vi "op_Pedestal.vi"(0 "EQ folder path Refnum":refnum<vi>, 1 "HV enable button":bool caption="High Voltage enable", 2 "HV parameters Refnum":refnum<vi>, 3 "HV level Refnum":refnum<vi>, 4 "HV string Refnum":refnum<vi>, 5 "Stop ACQ button Refnum":refnum<vi>, 6 "ACQ Parameters (cluster)":T2={"Acquisition Mode"=0, "Pulse width"=0, "DTP period"=1, "Number of events"=4000} caption="Acquisition Parameters" {"Number of events" min=1; "DTP period" min=1; "Pulse width" items=["25 ns", "50 ns", "75 ns", "100 ns"]; "Acquisition Mode" items=["Normal", "Pedestal", "Test Pulse", "Test Pulse trigger & synchronous"]}, 7 "Events to acquire Refnum":refnum<vi>, 8 "error tick Refnum":refnum<vi>, 9 "ACQ events fets Refnum":refnum<vi>, 10 "Operation text Refnum":refnum<vi>, 11 "ACQ events fets A Refnum":refnum<vi>, 12 "Busy Refnum":refnum<vi>, 13 "ACQ events fets B Refnum":refnum<vi>, 14 "Addresses Cluster":T1={"ENA1"=FALSE, "IP address 1"="172.16.14.22", "ENA2"=FALSE, "IP address 2"="172.16.14.23"}, 15 "etapa# terminals refnums":T3, 17 "GbReg params":u8[](array[numeric])=[32, 32]) -> (23 "Folder path: acquisition reports":path=path "C:/VIPauto/Files/LayerID/Acquisition/yyyymmdd_hh-mm-ss_Leak#_HV#")   [LabVIEW 2015, in "VIPM2.lvlib"]
uses:
  VIPM2.lvlib
panel:
  out "Chip ID list 2":u32[](array[numeric]) format="%.0x"
  out "Layer ID list 2 (ordered)":u32[](array[numeric]) format="%.0x"
  out "All ID list 2":u32[](array[numeric]) format="%.0x"
  out "All ID list 1":u32[](array[numeric]) format="%.0x"
  out "Layer ID list 1 (ordered)":u32[](array[numeric]) format="%.0x"
  out "Chip ID list 1":u32[](array[numeric]) format="%.0x"
  # "Operation: ACQuisition Pedestal with HV (refnums)"
  # "Analog Vref low"
  # "Gb THLD"
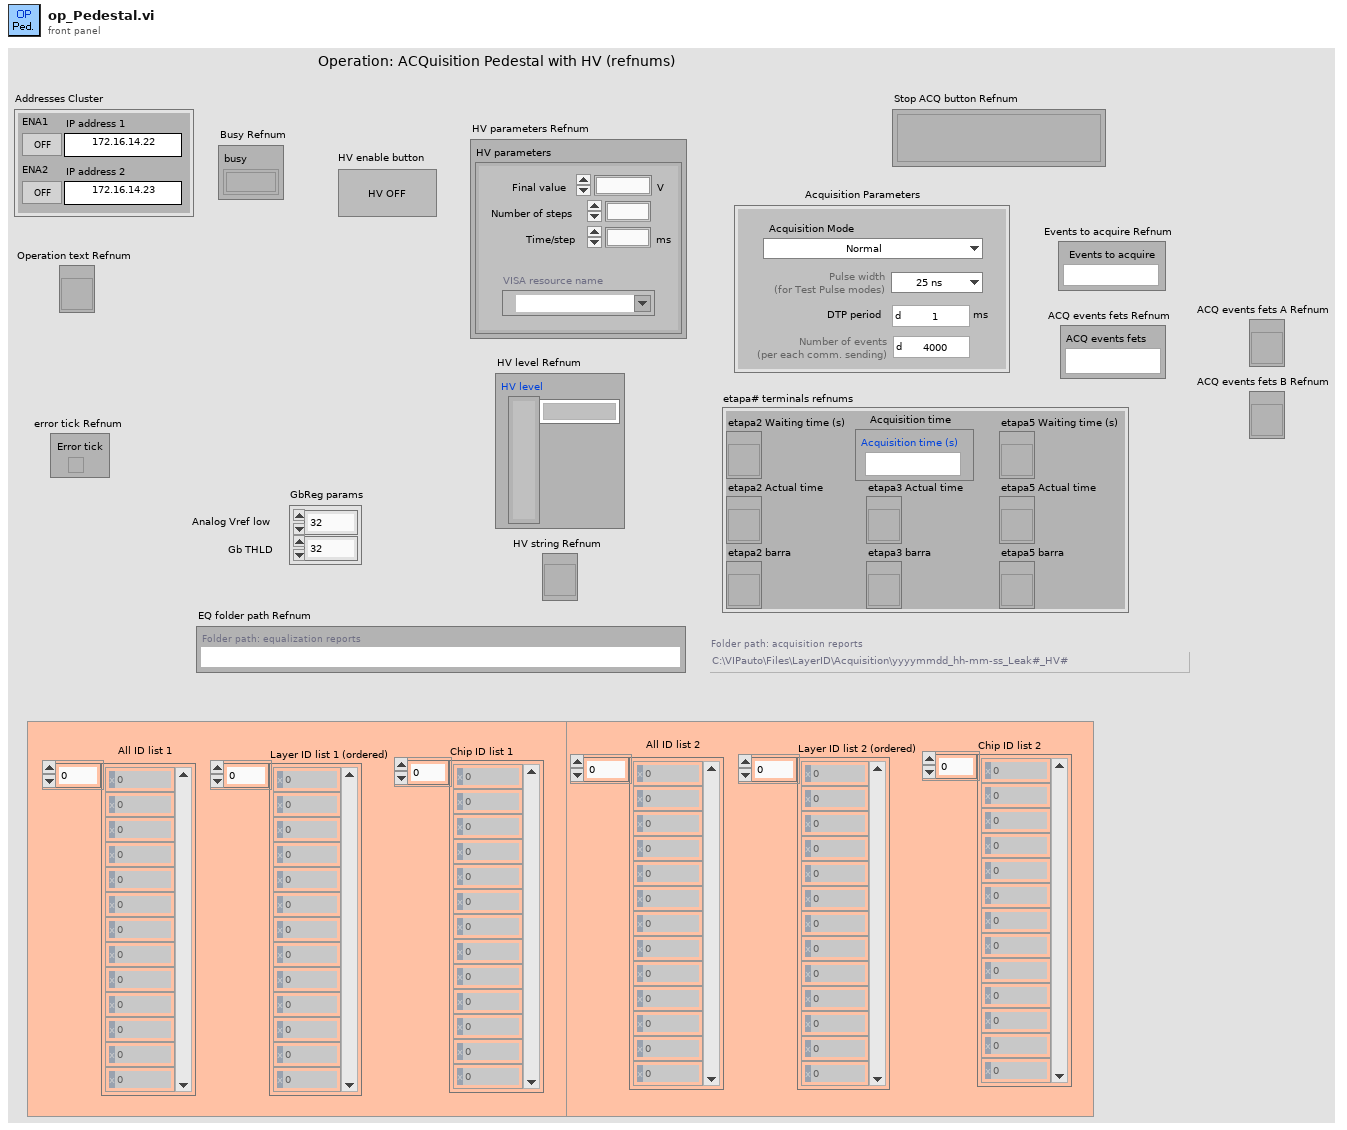
[diagram p1: front panel]
types:
  T1 = cluster{"ENA1":bool, "IP address 1":string, "ENA2":bool, "IP address 2":string}
  T2 = cluster{"Acquisition Mode":u32, "Pulse width":u32, "DTP period":u32, "Number of events":u32}
  T3 = cluster{"etapa2 Waiting time (s)":refnum<vi>, "etapa2 Actual time":refnum<vi>, "etapa2 barra":refnum<vi>, "etapa3 Actual time":refnum<vi>, "etapa3 barra":refnum<vi>, "etapa5 Waiting time (s)":refnum<vi>, "etapa5 Actual time":refnum<vi>, "etapa5 barra":refnum<vi>, "Acquisition time":refnum<vi>}
  T4 = enum8{"Enabled", "Disabled", "Disabled and Grayed Out"}
  T5 = cluster{"Final value":i16, "Number of steps":u8, "Time/step":u16, "Output Off Behavior":u16, "VISA resource name":refnum<visa-resource-name>}
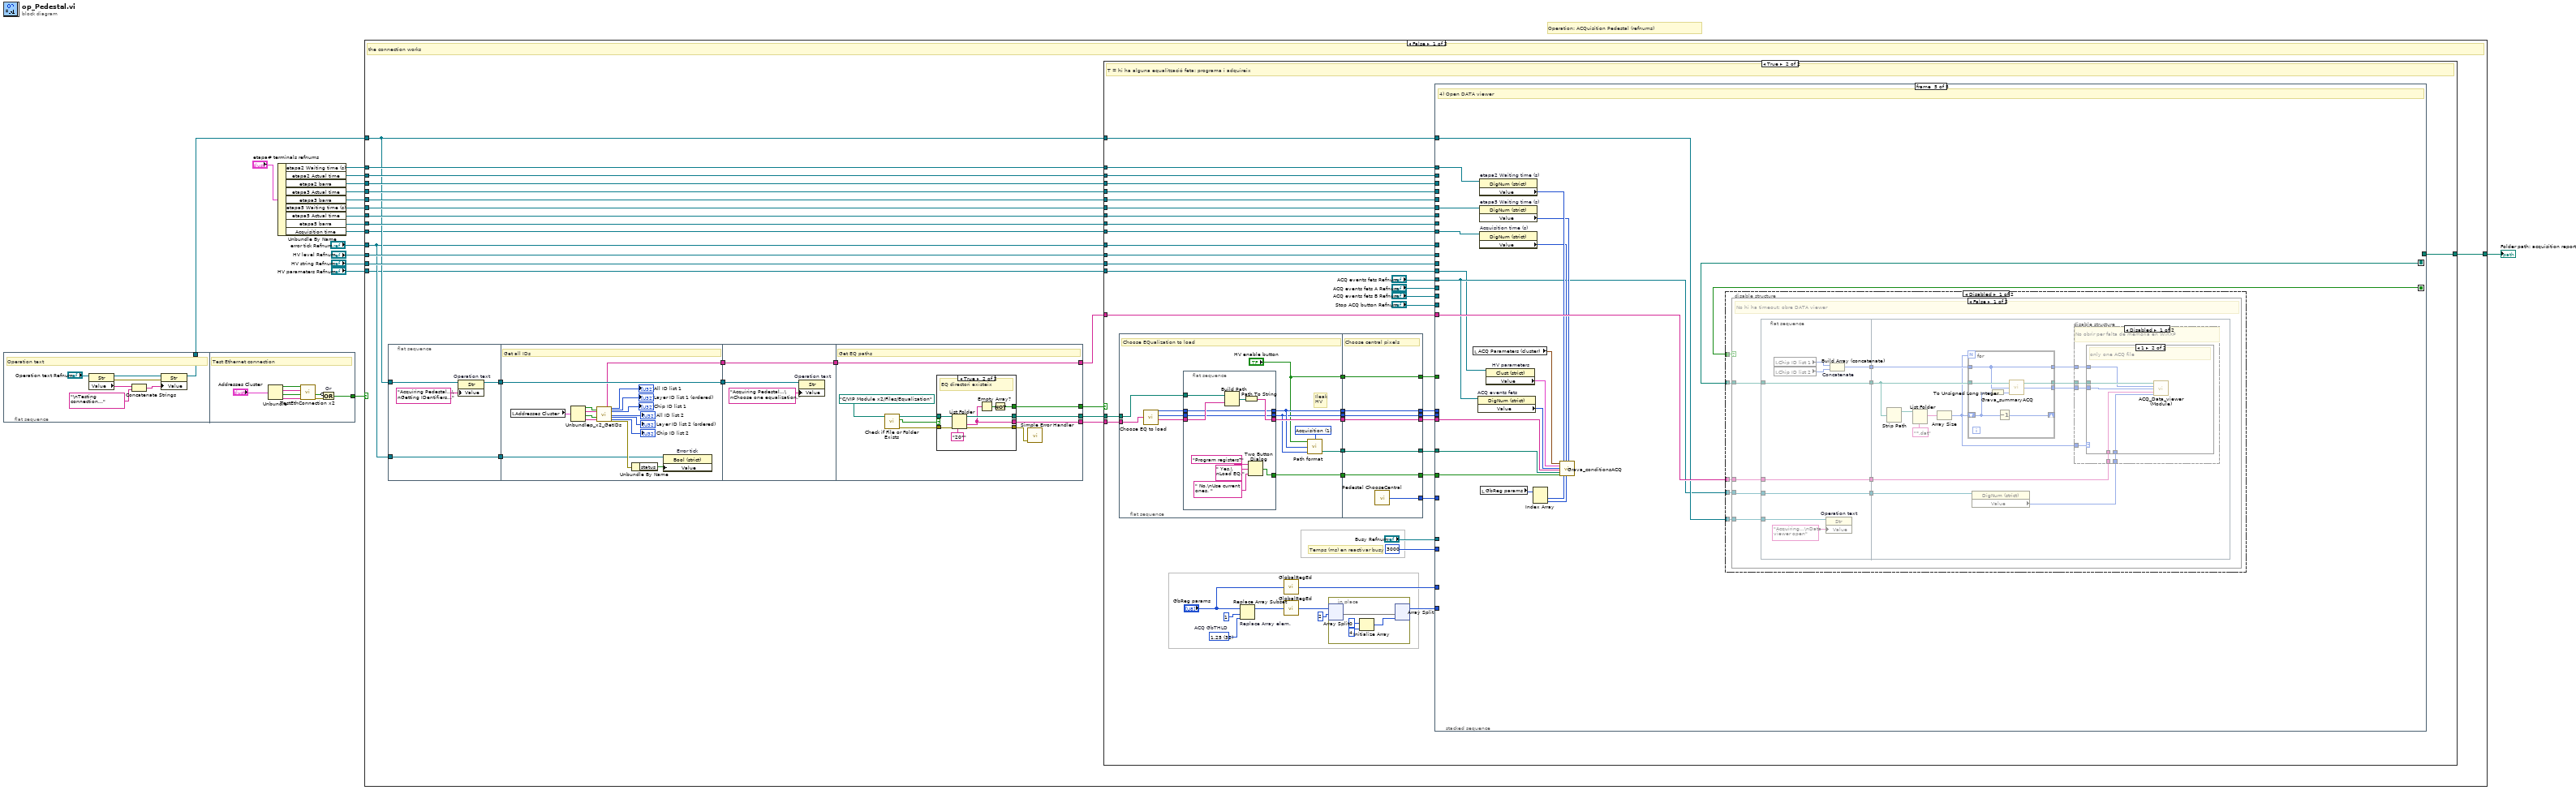
[diagram p0: block diagram]
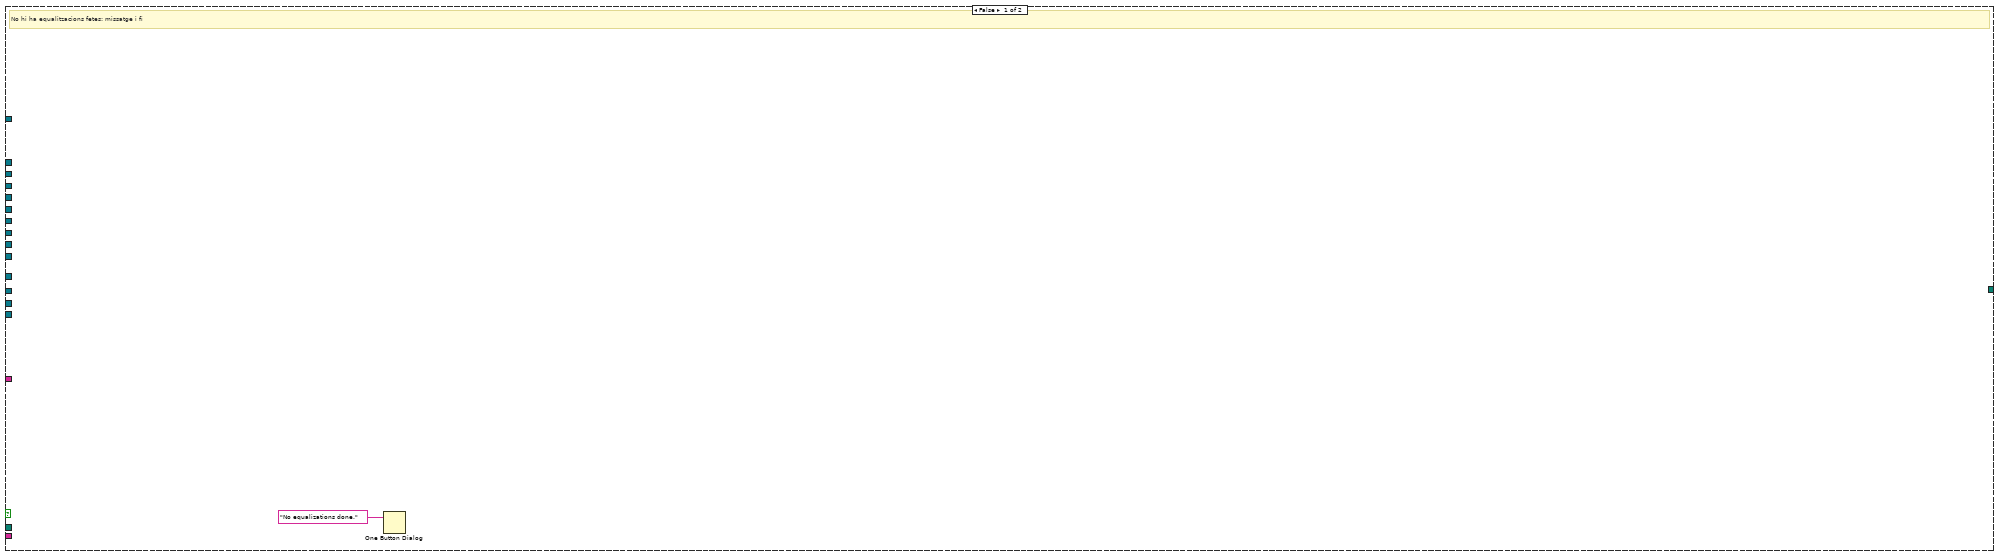
[diagram p3: hidden frame]
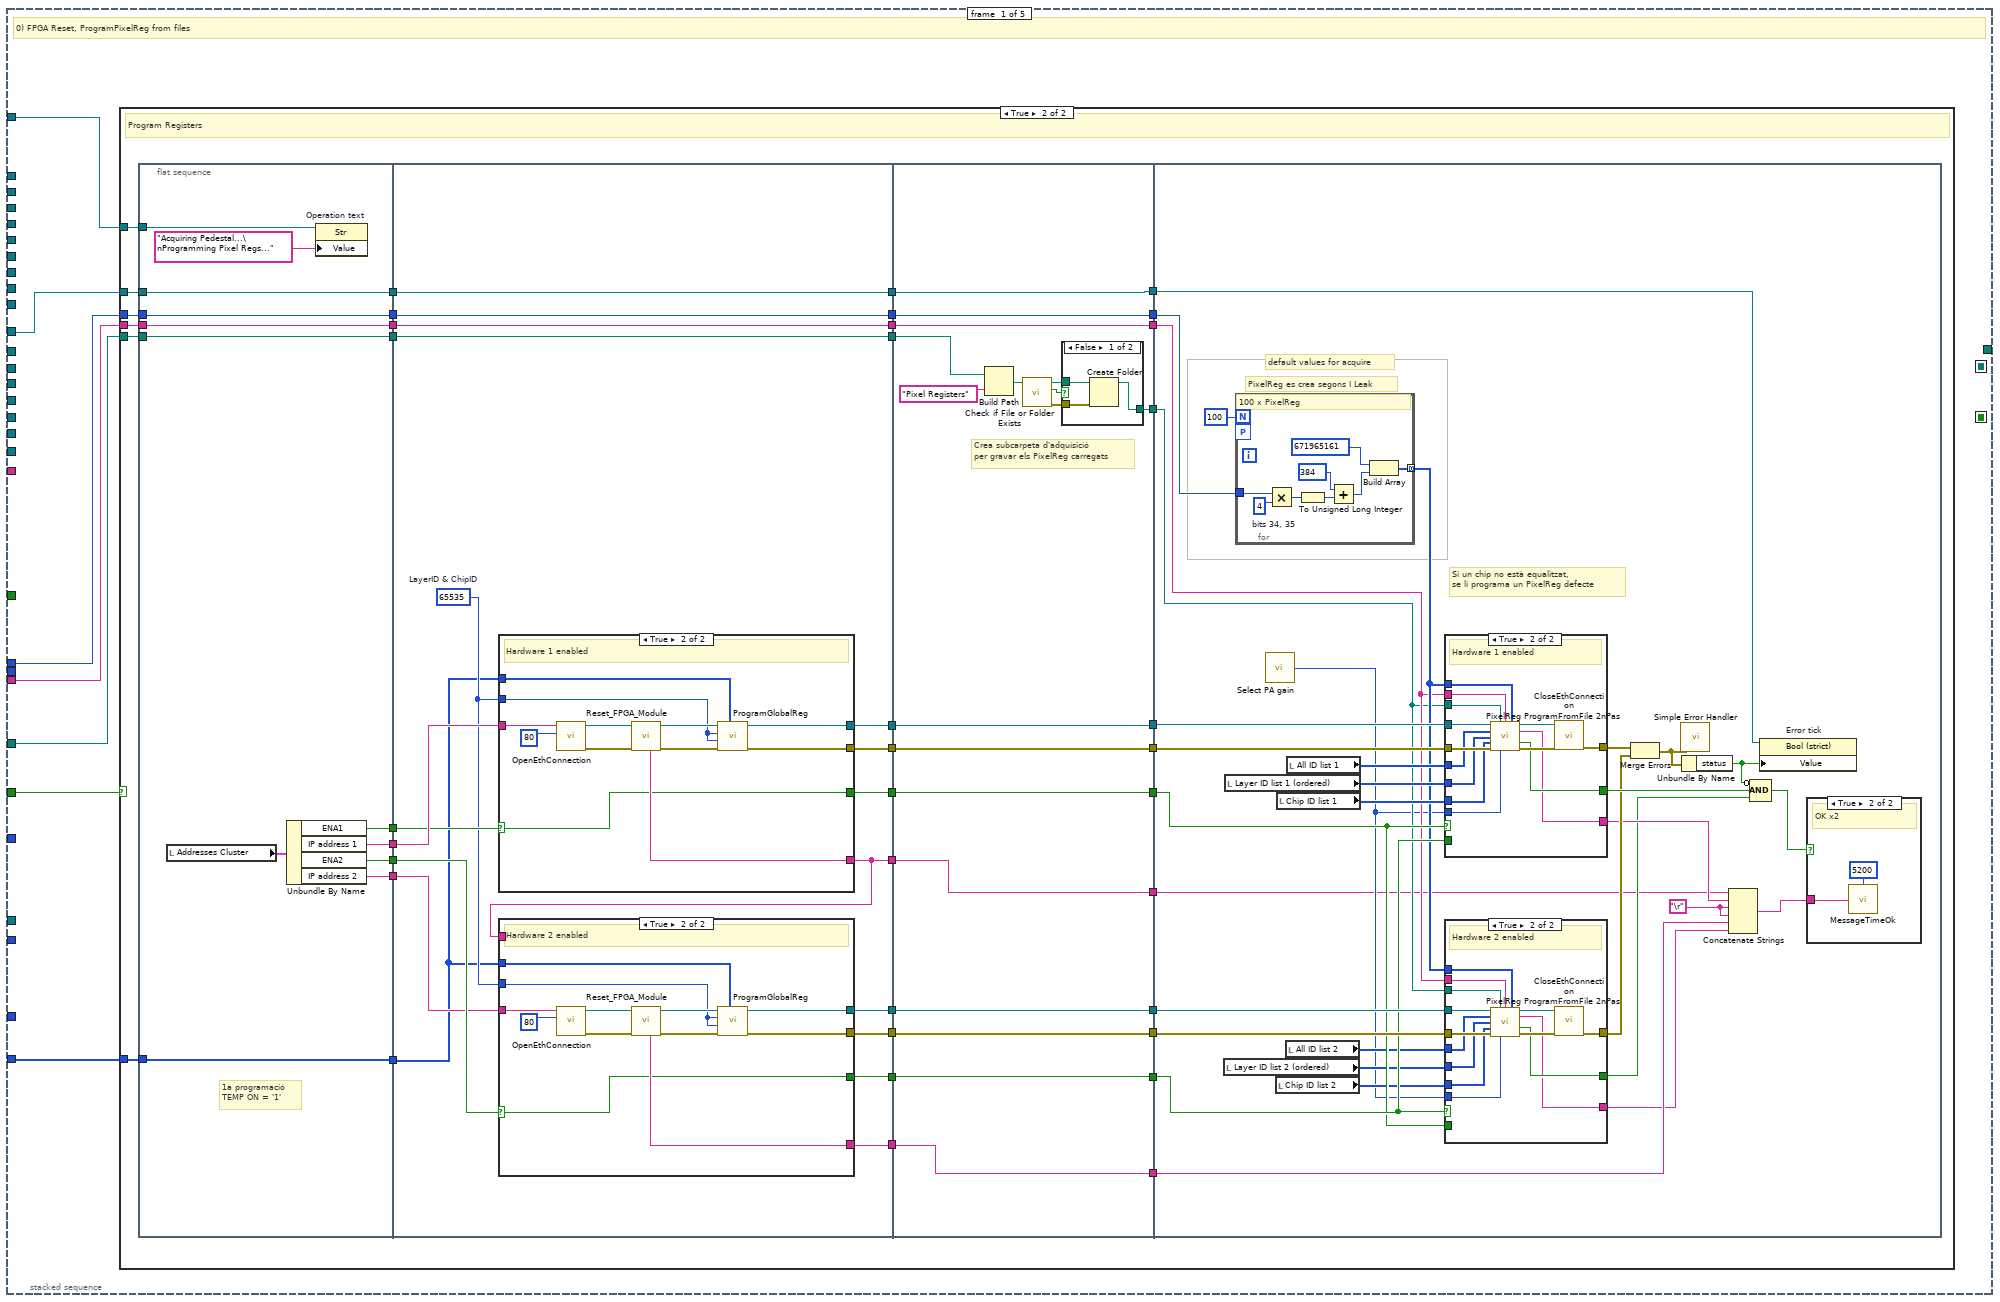
[diagram p4: hidden frame]
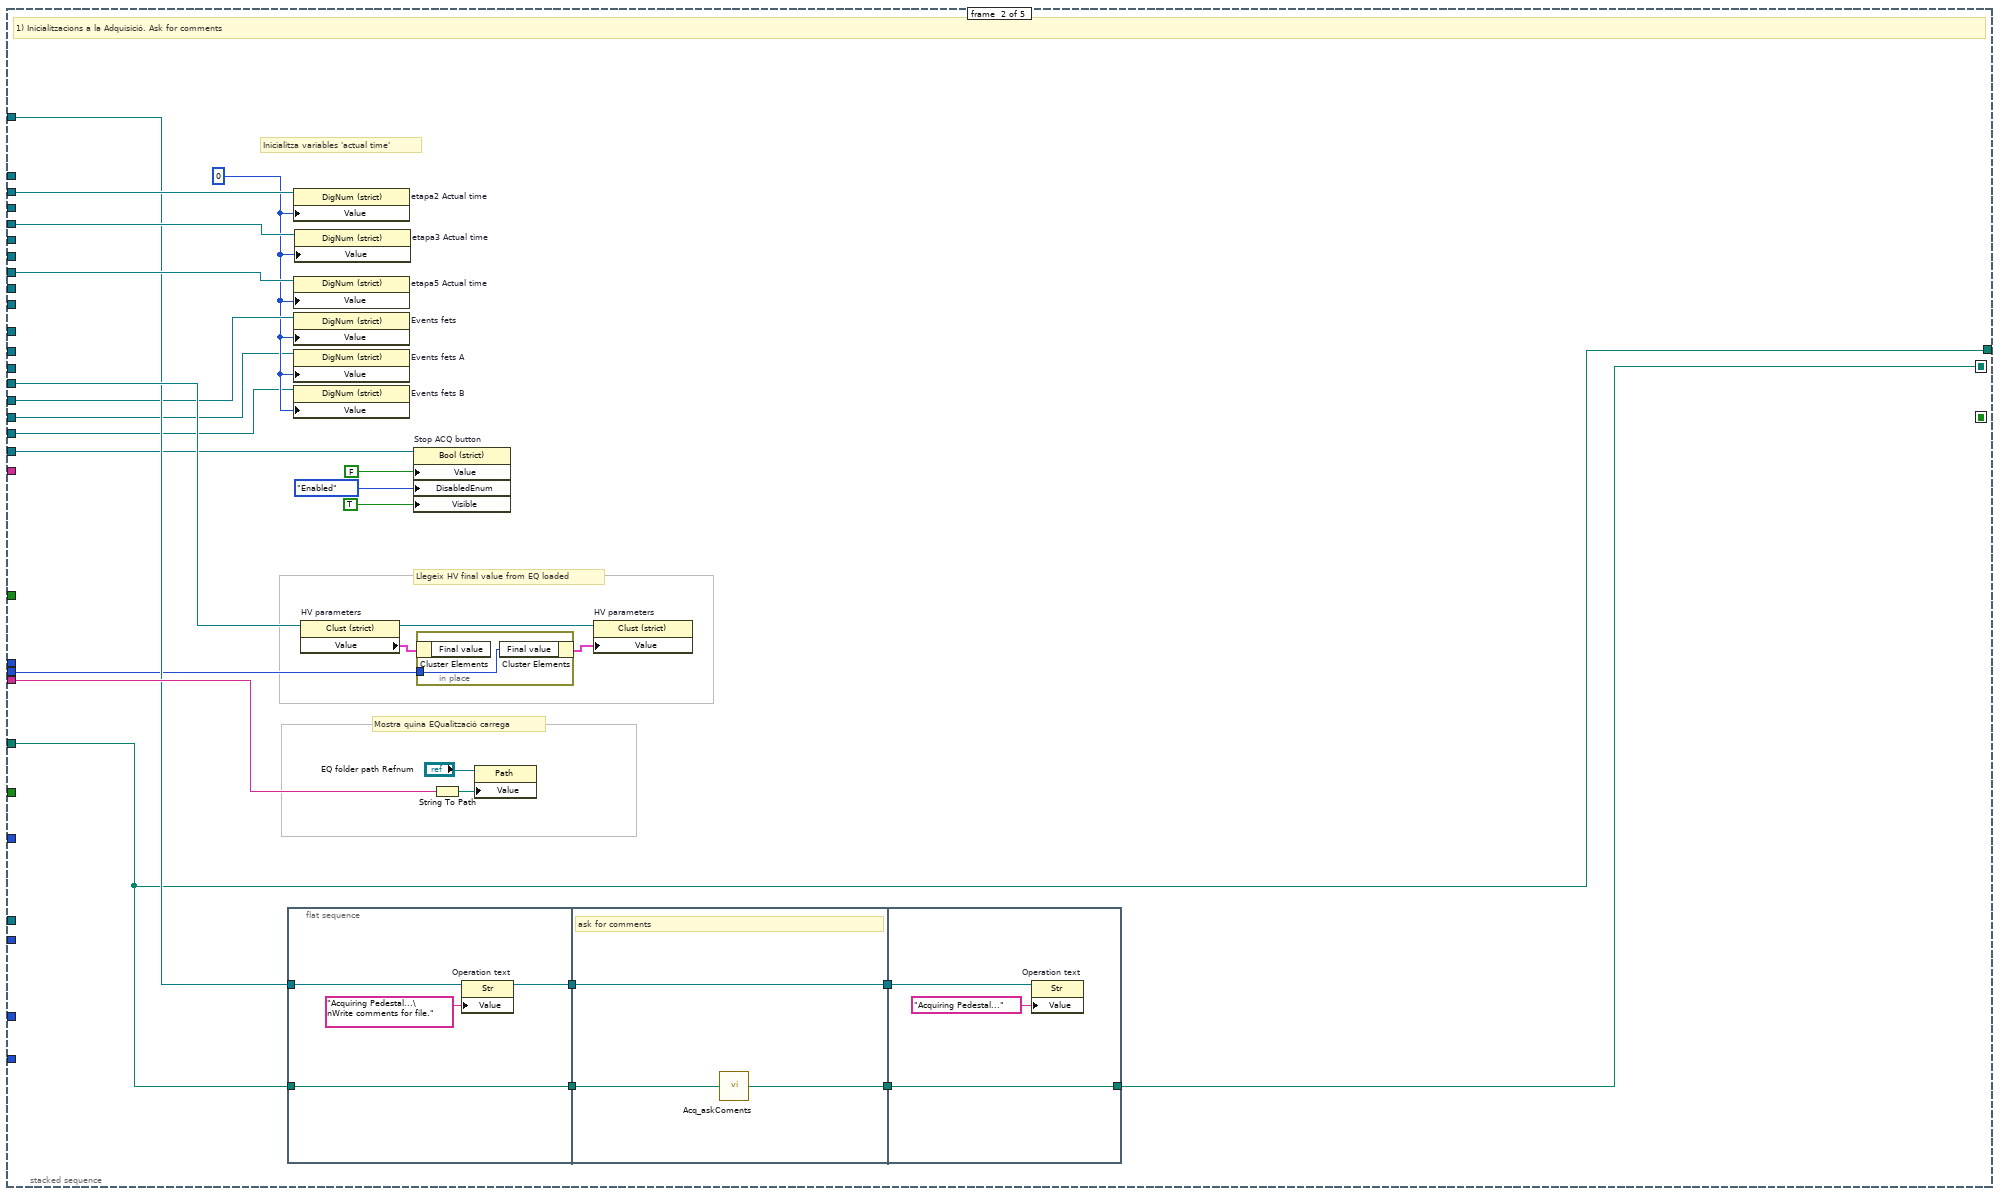
[diagram p12: hidden frame]
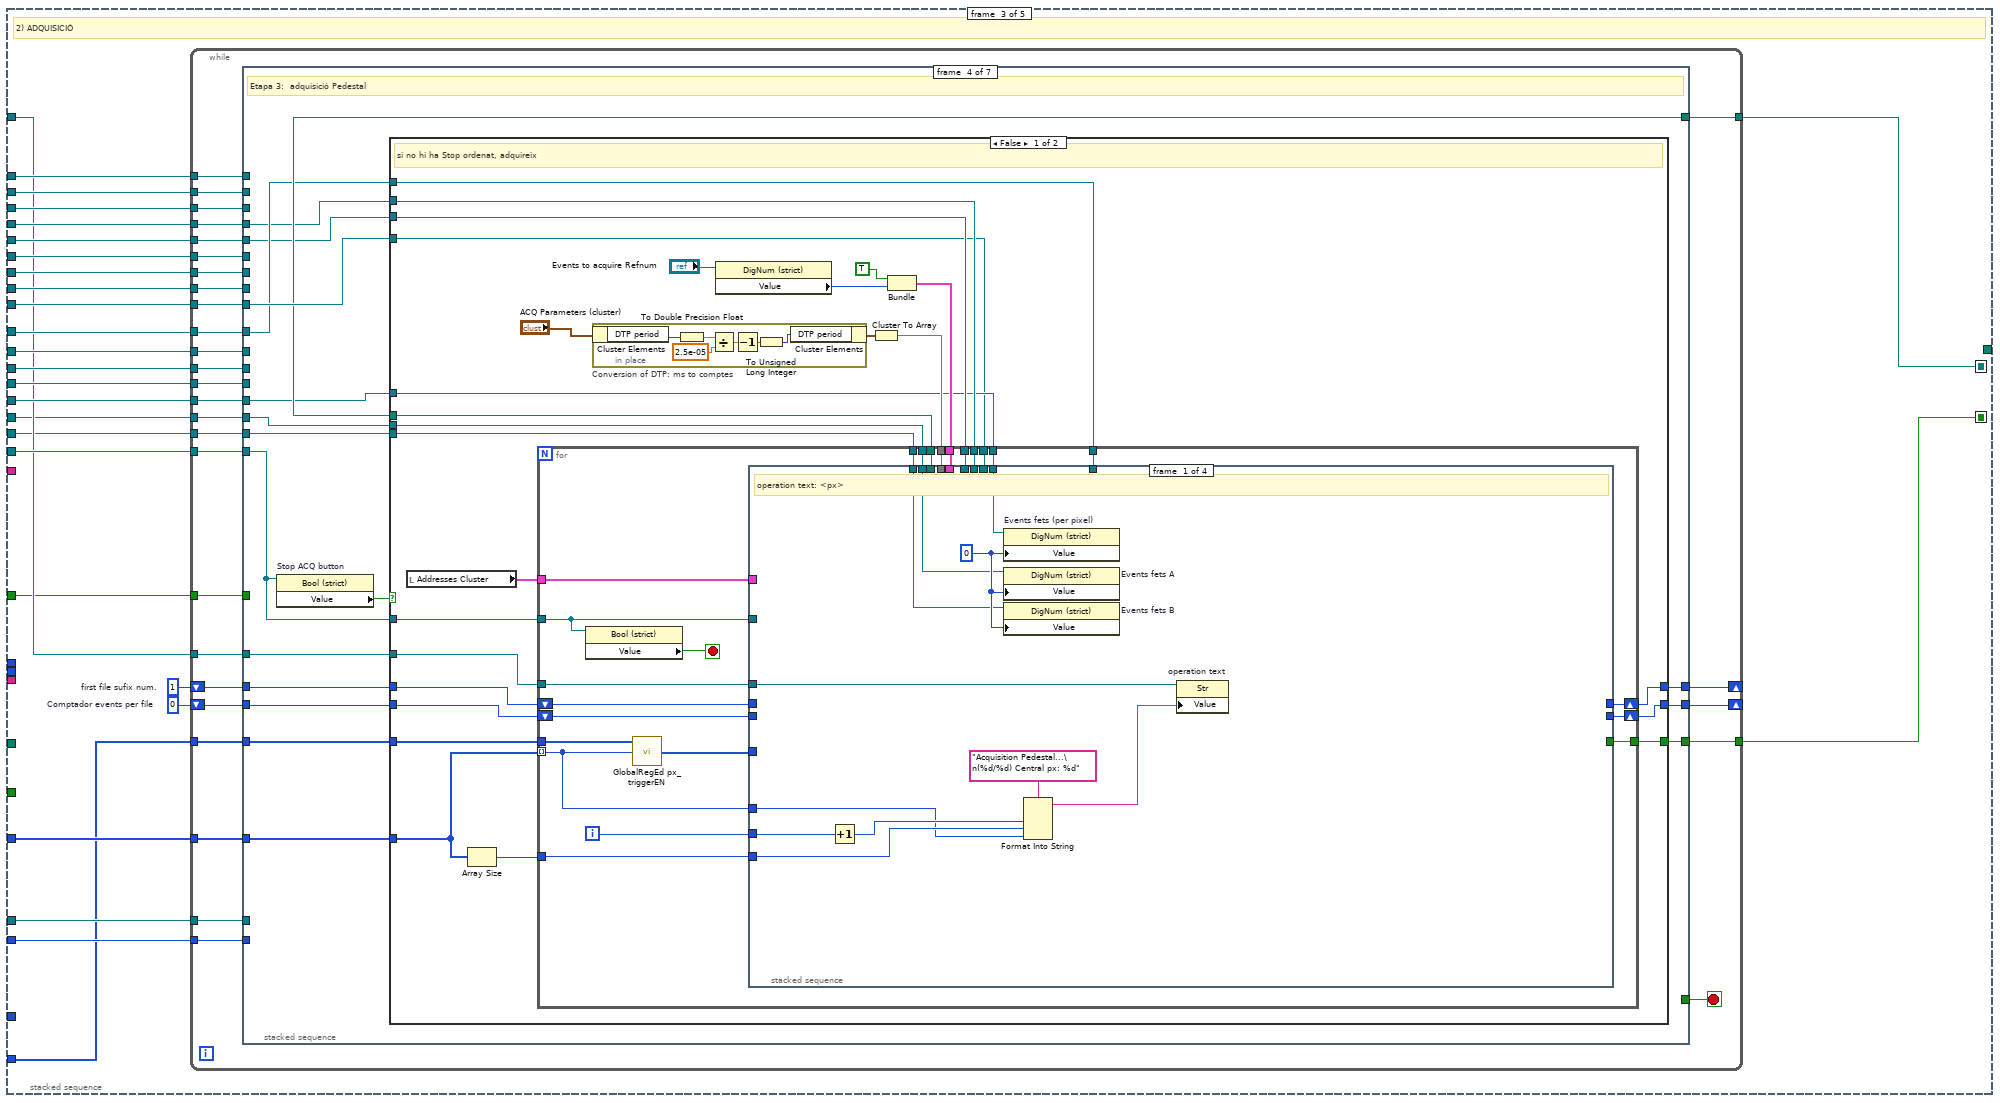
[diagram p13: hidden frame]
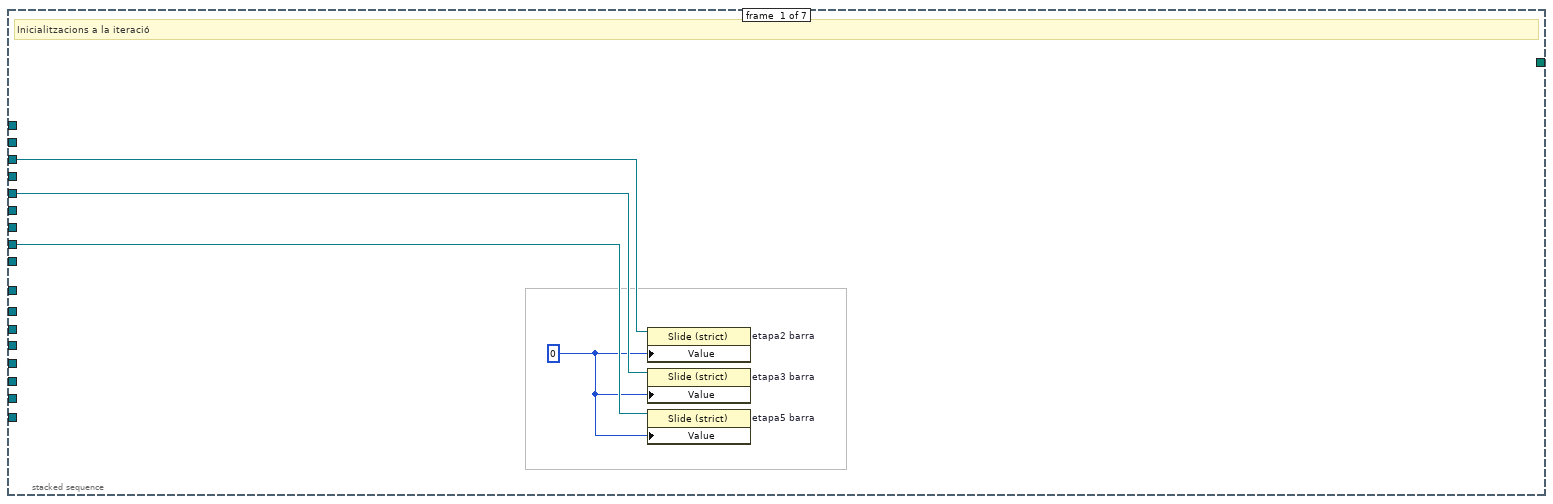
[diagram p14: hidden frame]
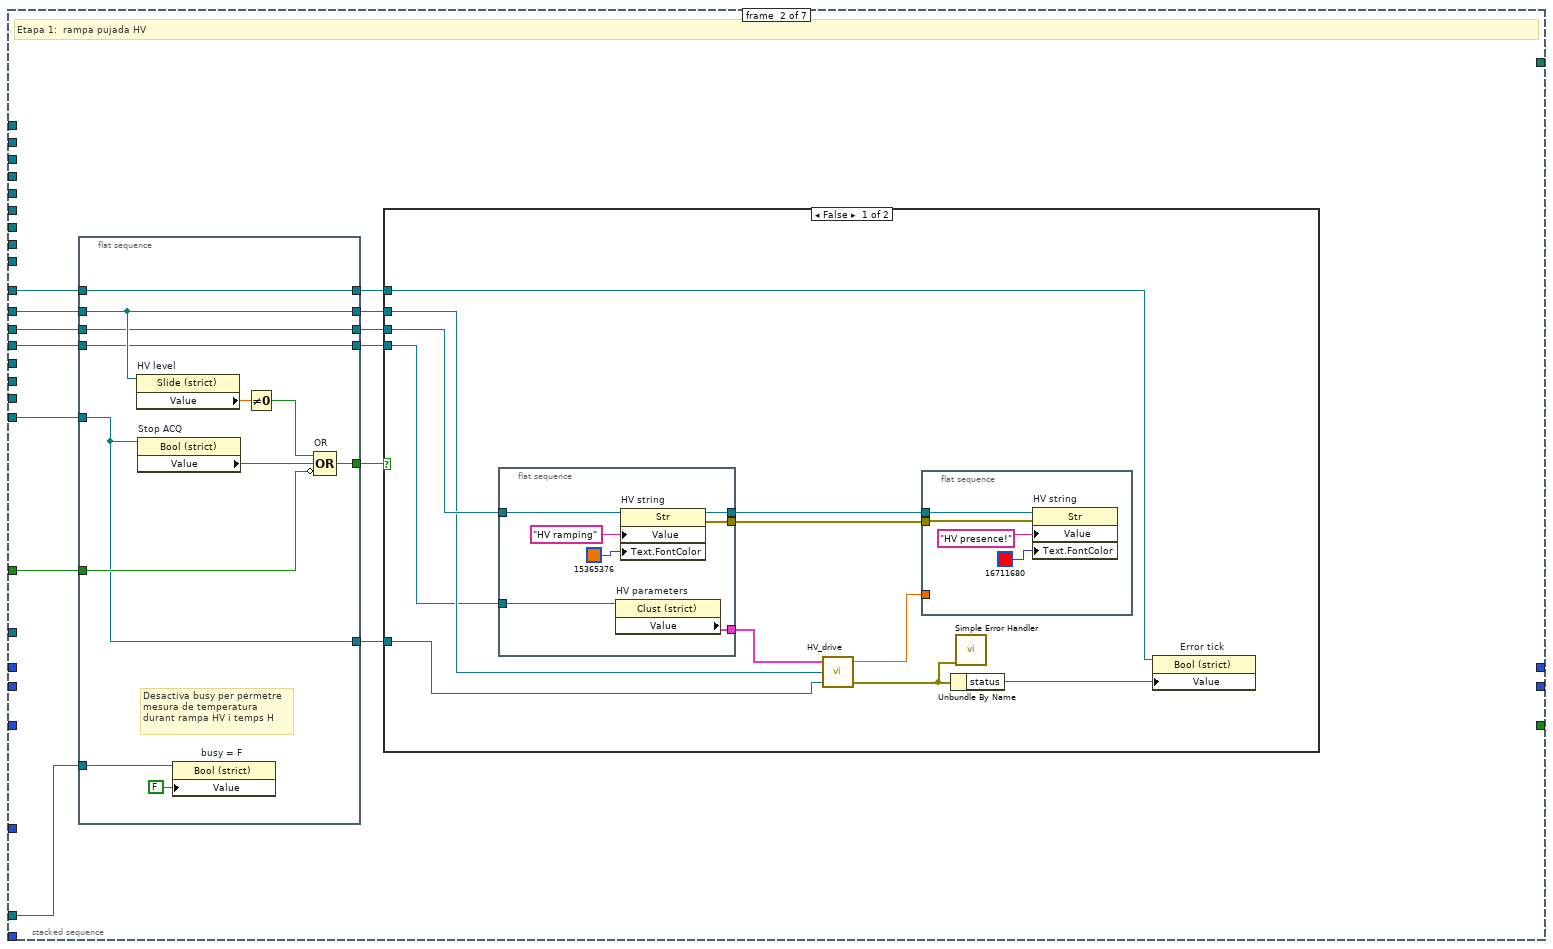
[diagram p15: hidden frame]
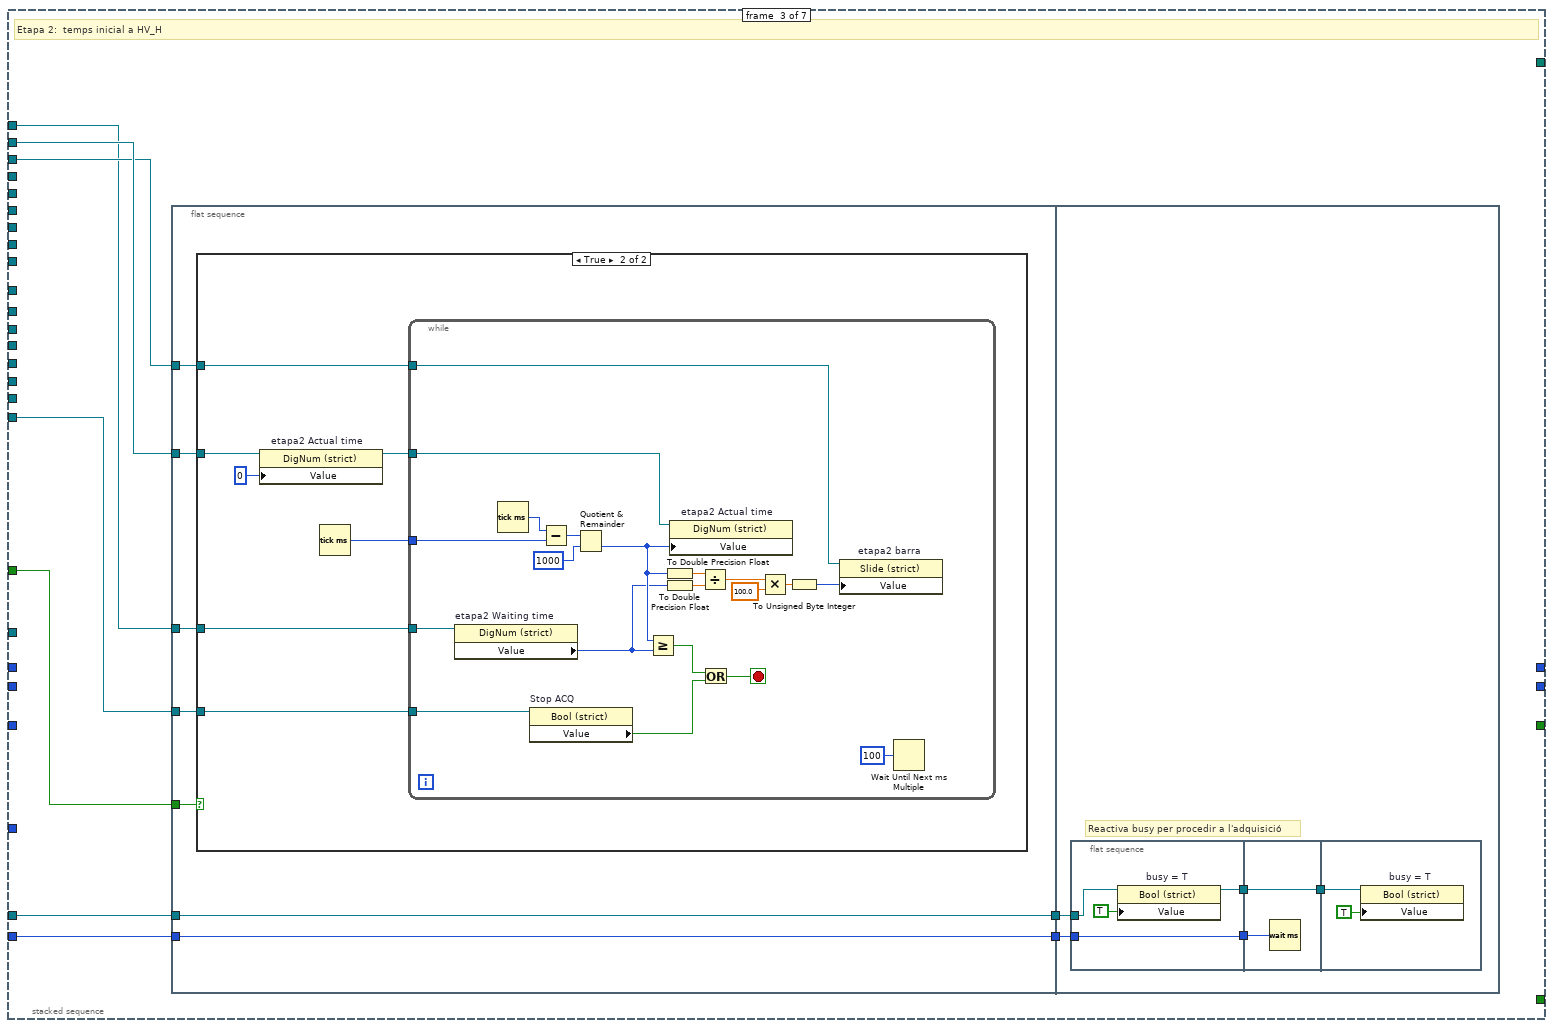
[diagram p17: hidden frame]
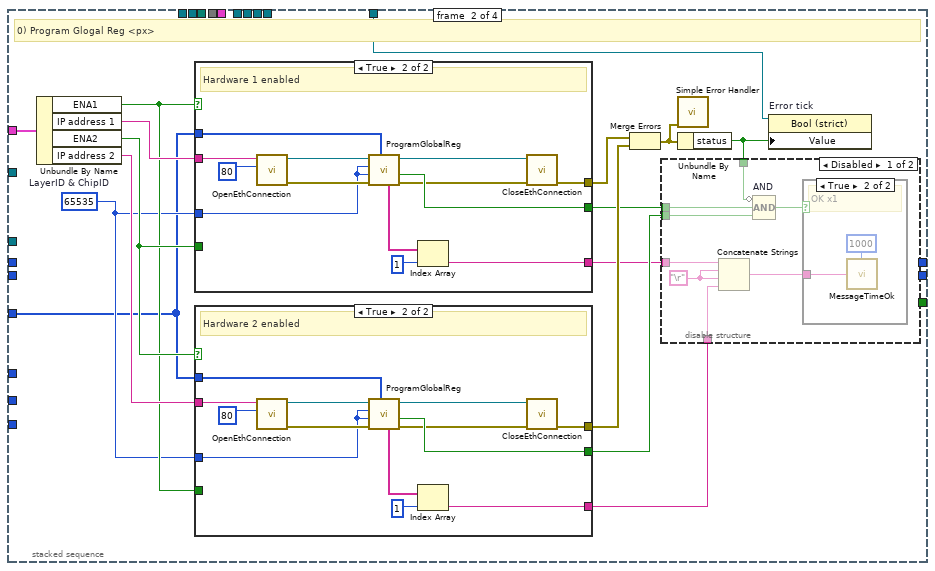
[diagram p19: hidden frame]
diagram:
  # "Operation: ACQuisition Pedestal (refnums)"
  n1 = flat-sequence {
    tunnel: [w18] -> w7
    tunnel: [w30] -> w17
    frame #0 {
      # "Operation text"
      n2 = property class="Str"(reference="Operation text Refnum") -> (reference out=w21:refnum<vi>, error out=w20:errorcluster, "Value"=w23:string)  [unwired: 1 in]
      n3 = Concatenate Strings "Concatenate Strings"(w23, "\nTesting connection..." ("string")) -> (w19:string)
      n4 = property class="Str"(reference=w21, error in=w20, "Value"=w19) -> (reference out=w18:refnum<vi>)  [unwired: 1 out]
    }
    frame #1 {
      # "Test Ethernet connection"
      n5 = Unbundle("Addresses Cluster") -> ("ENA1"=w28:bool, "IP address 1"=w27:string, "ENA2"=w26:bool, "IP address 2"=w25:string)
      n6 = call "TestEthConnection x2.vi"("IP address 2"=w25, "ENA2"=w26, "IP address 1"=w27, "ENA1"=w28) -> ("error out"=w31:errorcluster, "Answers OK?"=w32:bool)  [unwired: 6 in]
      n7 = Compound Arithmetic op=OR "Or"(invert w32, w31) -> (w30:bool)
    }
  }
  n8 = Unbundle By Name("etapa# terminals refnums") -> ("etapa2 Waiting time (s)"=w15:refnum<vi>, "etapa2 Actual time"=w14:refnum<vi>, "etapa2 barra"=w13:refnum<vi>, "etapa3 Actual time"=w12:refnum<vi>, "etapa3 barra"=w11:refnum<vi>, "etapa5 Waiting time (s)"=w10:refnum<vi>, "etapa5 Actual time"=w9:refnum<vi>, "etapa5 barra"=w8:refnum<vi>, "Acquisition time"=w2:refnum<vi>)
  n9 = case shown="False" w17 {
    selector: w17 -> [_ w1003]
    tunnel: w15 -> [w56 _]
    tunnel: w14 -> [w55 _]
    tunnel: w13 -> [w54 _]
    tunnel: w12 -> [w53 _]
    tunnel: w11 -> [w52 _]
    tunnel: w10 -> [w51 _]
    tunnel: w9 -> [w50 _]
    tunnel: w8 -> [w49 _]
    tunnel: w7 -> [w45 _]
    tunnel: "HV level Refnum" -> [w48 _]
    tunnel: "HV string Refnum" -> [w47 _]
    tunnel: "error tick Refnum" -> [w43 w1002]
    tunnel: [w46 _] -> w1
    tunnel: "HV parameters Refnum" -> [w37 _]
    tunnel: w2 -> [w36 _]
    frame False {
      # "the connection works"
      n10 = flat-sequence {
        tunnel: w45 -> [w60]
        tunnel: [w58] -> w44
        tunnel: w43 -> [w58]
        tunnel: [w57] -> w41
        tunnel: w44 -> [w74]
        tunnel: [w73] -> w42
        tunnel: w41 -> [w73]
        tunnel: [w72] -> w34
        tunnel: w42 -> [w78]
        tunnel: [w77] -> w35
        tunnel: w34 -> [w77]
        tunnel: [w84] -> w40
        tunnel: [w83] -> w39
        tunnel: [w82] -> w38
        tunnel: [w80] -> w33
        tunnel: w35 -> [w80]
        frame #0 {
          n11 = property on="Operation text" class="Str"(reference=w60, "Value"="Acquiring Pedestal...\nGetting IDentifiers...") -> (reference out=w57:refnum<vi>)  [unwired: 1 in, 1 out]
        }
        frame #1 {
          # "Get all IDs"
          n12 = local read "Addresses Cluster"() -> (w71:T1)
          n13 = Unbundle(w71) -> ("ENA1"=w70:bool, "IP address 1"=w69:string, "ENA2"=w67:bool, "IP address 2"=w68:string)
          n14 = call "op_x2_GetIDs.vi"("ENA1"=w70, "IP address 1"=w69, "ENA2"=w67, "IP address 2"=w68) -> ("summary IDs"=w72:string, "All ID list 1"=→"All ID list 1":u32[], "Layer ID list 1 (ordered)"=→"Layer ID list 1 (ordered)":u32[], "Chip ID list 1"=→"Chip ID list 1":u32[], "All ID list 2"=→"All ID list 2":u32[], "Layer ID list 2 (ordered)"=→"Layer ID list 2 (ordered)":u32[], "Chip ID list 2"=→"Chip ID list 2":u32[], "error out"=w75:errorcluster)  [unwired: 16 in]
          n15 = Unbundle By Name(w75) -> ("status"=w76:bool)
          n16 = property on="Error tick" class="Bool (strict)"(reference=w74, "Value"=w76) -> ()  [unwired: 1 in, 2 out]
        }
        frame #2 {
          n17 = property on="Operation text" class="Str"(reference=w78, "Value"="Acquiring Pedestal...\nChoose one equalization.") -> ()  [unwired: 1 in, 2 out]
        }
        frame #3 {
          # "Get EQ paths"
          n18 = call <vilib>:"Check if File or Folder Exists.vi"("path"=path "C:/VIP Module x2/Files/Equalization") -> ("error out"=w85:errorcluster, "file or folder exists?"=w86:bool, "dup path"=w87:path)  [unwired: 8 in]
          n19 = case shown="True" w86 {
            selector: w86 -> [w91 _]
            tunnel: w87 -> [w90 w97]
            tunnel: w85 -> [w89 w96]
            tunnel: [w91 w93] -> w84
            tunnel: [w90 w94] -> w83
            tunnel: [w89 w95] -> w81
            tunnel: [_ w92] -> w82
            frame False {
              # "no EQs"
            }
            frame True {
              # "EQ directori existeix"
              n20 = List Folder(path=w97, pattern="20*", error in=w96) -> (path out=w94:path, folder names=w92:string[], error out=w95:errorcluster)  [unwired: 1 in, 1 out]
              n21 = Empty Array?(array=w92) -> (empty?=w98:bool)
              n22 = Not(x=w98) -> (.not. x?=w93:bool)
            }
          }
          n23 = call <vilib>:"Simple Error Handler.vi"("error in (no error)"=w81) -> ()  [unwired: 4 in, 5 out]
        }
      }
      n24 = case shown="True" w40 {
        tunnel: w56 -> [_ w145]
        tunnel: w55 -> [_ w144]
        tunnel: w54 -> [_ w143]
        tunnel: w53 -> [_ w142]
        tunnel: w52 -> [_ w141]
        tunnel: w51 -> [_ w140]
        tunnel: w50 -> [_ w139]
        tunnel: w49 -> [_ w138]
        tunnel: w48 -> [_ w137]
        tunnel: w47 -> [_ w136]
        tunnel: [_ w135] -> w46
        tunnel: w45 -> [_ w134]
        tunnel: w43 -> [_ w133]
        tunnel: w39 -> [_ w132]
        tunnel: w38 -> [_ w131]
        tunnel: w37 -> [_ w127]
        tunnel: w36 -> [_ w124]
        tunnel: w33 -> [_ w122]
        frame False {
          # "No hi ha equalitzacions fetes: missatge i fi"
          n25 = One Button Dialog(message="No equalizations done.") -> ()  [unwired: 1 in, 1 out]
        }
        frame True {
          w107 = u8 32 items=["0.34", "0.37", "0.40", "0.43", "0.45", "0.48", "0.51", "0.54", "0.57", "0.60", "0.63", "0.65", "0.68", "0.71", "0.74", "0.77", "0.80", "0.82", "0.85", "0.88", "0.91", "0.94", "0.97", "0.99", "1.02", "1.05", "1.08", "1.11", "1.14", "1.16", "1.19", "1.22", "1.25", "1.28", "1.31", "1.34", "1.36", "1.39", "1.42", "1.45", "1.48", "1.51", "1.53", "1.56", "1.59", "1.62", "1.65", "1.68", "1.70", "1.73", "1.76", "1.79", "1.82", "1.85", "1.88", "1.90", "1.93", "1.96", "1.99", "2.02", "2.05", "2.07", "2.10", "2.13"]  # ACQ GbTHLD
          # "Temps (ms) en reactivar busy"
          # "T = hi ha alguna equalització feta: programa i adquireix"
          n26 = flat-sequence {
            tunnel: w132 -> [w158]
            tunnel: w131 -> [w159]
            tunnel: [w156] -> w117
            tunnel: [w151] -> w116
            tunnel: [w154] -> w115
            tunnel: [w160] -> w114
            tunnel: [w155] -> w113
            tunnel: ["HV enable button"] -> w112
            tunnel: [w173] -> w118
            tunnel: [w174] -> w121
            tunnel: [w175] -> w126
            tunnel: [w176] -> w128
            tunnel: [w177] -> w129
            tunnel: [w178] -> w130
            tunnel: w117 -> [w178]
            tunnel: w116 -> [w177]
            tunnel: w115 -> [w176]
            tunnel: w114 -> [w175]
            tunnel: w113 -> [w174]
            tunnel: w112 -> [w173]
            tunnel: [w172] -> w111
            frame #0 {
              w161 = u8 1 items=["Equalization", "Acquisition"] ("Operation type")
              # "Ileak\nHV"
              # "Choose EQualization to load"
              n27 = call "Choose EQ to load.vi"("EQ folders"=w159) -> ("I Leakage"=w153:u8, "HV last value"=w152:i16, "loaded EQ folder"=w157:string)  [unwired: 5 in]
              n28 = flat-sequence {
                tunnel: w158 -> [w171]
                tunnel: w157 -> [w170]
                tunnel: [w168] -> w156
                tunnel: [w167] -> w155
                tunnel: [w163] -> w154
                tunnel: w153 -> [w163]
                tunnel: w152 -> [w162]
                tunnel: [w162] -> w151
                frame #0 {
                  n29 = Build Path(base path=w171, name or relative path=w170) -> (appended path=w169:path)
                  n30 = Path To String(path=w169) -> (string=w168:string)
                  n31 = Two Button Dialog(message="Program registers?", 1:" No.\nUse current ones. " ("F button name (\"Cancel\")"), 2:" Yes.\nLoad EQ." ("T button name (\"OK\")")) -> (T button?=w167:bool)
                }
              }
              n32 = call "Path format.vi"("Operation type"=w161, "HV level"=w151, "I leakage"=w154, "HV enable button"="HV enable button") -> ("folder path"=w160:path)  [unwired: 1 in]
            }
            frame #1 {
              # "Choose central pixels"
              n33 = call "Pedestal ChooseCentral.vi"() -> ("Central pixels"=w172:u8[])  [unwired: 5 in]
            }
          }
          n34 = Replace Array Subset "Replace Array elem."(array="GbReg params", new element=w107, index=1) -> (w106:u8[])
          n35 = call "GlobalRegEd.vi"("params"="GbReg params") -> ("Global Reg out"=w101:u32[])  [unwired: 4 in]
          n36 = call "GlobalRegEd.vi"("params"=w106) -> ("Global Reg out"=w105:u32[])  [unwired: 4 in]
          n37 = in-place {
            n38 = in-place-split #1(w105, 2) -> (w149:u32[])  [unwired: 1 out]
            n39 = Initialize Array "Initialize Array"(u32 0, 4 ("dimension size")) -> (w146:u32[])
            n40 = in-place-split #1(w149, w146) -> (w103:u32[])  [unwired: 1 out]
          }
          n41 = stacked-sequence {
            seq-local: [_ _ w425 _ _] -> [_ _ _ _ w948]
            seq-local: [_ w387 _ _ _] -> [_ _ w426 _ w947]
            tunnel: w134 -> [w185 w392 w421 w868 w945]
            tunnel: w145 -> [_ _ w440 _ w928]
            tunnel: w144 -> [_ w402 w439 _ _]
            tunnel: w143 -> [_ _ w438 _ _]
            tunnel: w142 -> [_ w401 w437 _ _]
            tunnel: w141 -> [_ _ w436 _ _]
            tunnel: w140 -> [_ _ w435 _ w929]
            tunnel: w139 -> [_ w400 w434 _ _]
            tunnel: w138 -> [_ _ w433 _ _]
            tunnel: w133 -> [w184 _ w430 w870 _]
            tunnel: w137 -> [_ _ w432 _ _]
            tunnel: w136 -> [_ _ w431 _ _]
            tunnel: [_ w385 _ _ _] -> w135
            tunnel: w130 -> [w183 w393 _ _ w933]
            tunnel: w129 -> [_ w391 _ _ _]
            tunnel: w128 -> [w182 _ _ _ _]
            tunnel: w127 -> [_ w399 w429 _ w931]
            tunnel: w126 -> [w181 w385 _ _ w934]
            tunnel: "Stop ACQ button Refnum" -> [_ w384 w428 w867 _]
            tunnel: w124 -> [_ _ w427 _ w930]
            tunnel: "ACQ events fets Refnum" -> [_ w380 w424 _ w932]
            tunnel: w122 -> [_ _ _ _ w946]
            tunnel: w121 -> [w180 _ _ _ w935]
            tunnel: "Busy Refnum" -> [_ _ w423 w866 _]
            tunnel: u32 3000 -> [_ _ w422 _ _]
            tunnel: w118 -> [_ _ w420 _ _]
            tunnel: w111 -> [_ _ w419 _ _]
            tunnel: "ACQ events fets A Refnum" -> [_ w378 w418 _ _]
            tunnel: "ACQ events fets B Refnum" -> [_ w377 w417 _ _]
            tunnel: w103 -> [w179 _ w414 _ _]
            tunnel: w101 -> [_ _ _ w865 _]
            frame #0 {
              # "0) FPGA Reset, ProgramPixelReg from files"
              n42 = case shown="True" w180 {
                tunnel: w185 -> [_ w211]
                tunnel: w184 -> [_ w210]
                tunnel: w183 -> [_ w209]
                tunnel: w182 -> [_ w208]
                tunnel: w181 -> [_ w207]
                tunnel: w179 -> [_ w186]
                frame False {
                  # "Use current registers values"
                }
                frame True {
                  # "Program Registers"
                  n43 = flat-sequence {
                    tunnel: w211 -> [w235]
                    tunnel: [w234] -> w224
                    tunnel: w210 -> [w234]
                    tunnel: [w233] -> w223
                    tunnel: w209 -> [w233]
                    tunnel: [w232] -> w222
                    tunnel: w208 -> [w232]
                    tunnel: [w231] -> w221
                    tunnel: w207 -> [w231]
                    tunnel: [w229] -> w206
                    tunnel: [w228] -> w205
                    tunnel: [w227] -> w204
                    tunnel: [w226] -> w203
                    tunnel: [w225] -> w187
                    tunnel: w186 -> [w225]
                    tunnel: [w254] -> w220
                    tunnel: w224 -> [w254]
                    tunnel: w223 -> [w253]
                    tunnel: [w253] -> w219
                    tunnel: w222 -> [w252]
                    tunnel: [w252] -> w218
                    tunnel: w221 -> [w251]
                    tunnel: [w251] -> w217
                    tunnel: w206 -> [w246]
                    tunnel: w205 -> [w241]
                    tunnel: w204 -> [w247]
                    tunnel: w203 -> [w240]
                    tunnel: [w248] -> w202
                    tunnel: [w249] -> w201
                    tunnel: [w250] -> w200
                    tunnel: [w237] -> w199
                    tunnel: [w245] -> w198
                    tunnel: [w244] -> w197
                    tunnel: [w243] -> w196
                    tunnel: [w242] -> w195
                    tunnel: w187 -> [w238]
                    tunnel: [w288] -> w216
                    tunnel: [w287] -> w215
                    tunnel: [w298] -> w214
                    tunnel: w220 -> [w298]
                    tunnel: [w297] -> w213
                    tunnel: w219 -> [w297]
                    tunnel: [w296] -> w212
                    tunnel: w218 -> [w296]
                    tunnel: w217 -> [w290]
                    tunnel: w202 -> [w288]
                    tunnel: w201 -> [w287]
                    tunnel: w200 -> [w286]
                    tunnel: w199 -> [w282]
                    tunnel: w198 -> [w285]
                    tunnel: w197 -> [w284]
                    tunnel: w196 -> [w283]
                    tunnel: w195 -> [w281]
                    tunnel: [w289] -> w194
                    tunnel: [w286] -> w193
                    tunnel: [w285] -> w192
                    tunnel: [w284] -> w191
                    tunnel: [w283] -> w190
                    tunnel: [w282] -> w189
                    tunnel: [w281] -> w188
                    tunnel: w216 -> [w329]
                    tunnel: w215 -> [w328]
                    tunnel: w214 -> [w331]
                    tunnel: w213 -> [w311]
                    tunnel: w212 -> [w326]
                    tunnel: w194 -> [w310]
                    tunnel: w193 -> [w319]
                    tunnel: w192 -> [w322]
                    tunnel: w191 -> [w321]
                    tunnel: w190 -> [w320]
                    tunnel: w189 -> [w304]
                    tunnel: w188 -> [w307]
                    frame #0 {
                      # "1a programació\nTEMP ON = '1'"
                      n44 = local read "Addresses Cluster"() -> (w230:T1)
                      n45 = Unbundle By Name(w230) -> ("ENA1"=w229:bool, "IP address 1"=w227:string, "ENA2"=w228:bool, "IP address 2"=w226:string)
                      n46 = property on="Operation text" class="Str"(reference=w235, "Value"="Acquiring Pedestal...\nProgramming Pixel Regs...") -> ()  [unwired: 1 in, 2 out]
                    }
                    frame #1 {
                      w239 = u32 65535  # LayerID & ChipID
                      n47 = case shown="True" w246 {
                        selector: w246 -> [w268 w269]
                        tunnel: w239 -> [_ w271]
                        tunnel: [_ w275] -> w248
                        tunnel: [_ w274] -> w249
                        tunnel: [_ w273] -> w237
                        tunnel: w238 -> [_ w272]
                        tunnel: w247 -> [_ w270]
                        tunnel: [w268 w269] -> w250
                        frame False {
                          # "Hardware 1 not enabled"
                        }
                        frame True {
                          # "Hardware 1 enabled"
                          n48 = call "OpenEthConnection.vi"("Port"=u16 80, "IP address"=w270) -> ("error out"=w279:errorcluster, "connection ID out"=w280:refnum<k5>)  [unwired: 7 in, 1 out]
                          n49 = call "Reset_FPGA_Module.vi"("error in (no error)"=w279, "connection ID"=w280) -> ("error out"=w276:errorcluster, "connection ID out"=w277:refnum<k5>, "Answer to Reset"=w273:string)  [unwired: 7 in]
                          n50 = call "ProgramGlobalReg.vi"("Global Reg"=w272, "error in (no error)"=w276, "ChipID"=w271, "LayerID"=w271, "connection ID"=w277) -> ("error out"=w274:errorcluster, "connection ID out"=w275:refnum<k5>)  [unwired: 2 in, 3 out]
                        }
                      }
                      n51 = case shown="True" w241 {
                        selector: w241 -> [w255 w256]
                        tunnel: w239 -> [_ w258]
                        tunnel: [_ w262] -> w245
                        tunnel: [_ w261] -> w244
                        tunnel: [_ w260] -> w242
                        tunnel: w238 -> [_ w259]
                        tunnel: w240 -> [_ w257]
                        tunnel: [w255 w256] -> w243
                        tunnel: w237 -> [_ _]
                        frame False {
                          # "Hardware 2 not enabled"
                        }
                        frame True {
                          # "Hardware 2 enabled"
                          n52 = call "OpenEthConnection.vi"("Port"=u16 80, "IP address"=w257) -> ("error out"=w266:errorcluster, "connection ID out"=w267:refnum<k5>)  [unwired: 7 in, 1 out]
                          n53 = call "Reset_FPGA_Module.vi"("error in (no error)"=w266, "connection ID"=w267) -> ("error out"=w263:errorcluster, "connection ID out"=w264:refnum<k5>, "Answer to Reset"=w260:string)  [unwired: 7 in]
                          n54 = call "ProgramGlobalReg.vi"("Global Reg"=w259, "error in (no error)"=w263, "ChipID"=w258, "LayerID"=w258, "connection ID"=w264) -> ("error out"=w261:errorcluster, "connection ID out"=w262:refnum<k5>)  [unwired: 2 in, 3 out]
                        }
                      }
                    }
                    frame #2 {
                      # "Crea subcarpeta d'adquisició\nper gravar els PixelReg carregats"
                      n55 = Build Path(base path=w290, name or relative path="Pixel Registers") -> (appended path=w294:path)
                      n56 = call <vilib>:"Check if File or Folder Exists.vi"("path"=w294) -> ("error out"=w291:errorcluster, "file or folder exists?"=w293:bool, "dup path"=w292:path)  [unwired: 8 in]
                      n57 = case shown="False" w293 {
                        tunnel: w292 -> [w301 w302]
                        tunnel: w291 -> [w300 _]
                        tunnel: [w299 w302] -> w289
                        frame False {
                          n58 = Create Folder(path (use dialog)=w301, error in=w300) -> (created path=w299:path)  [unwired: 1 in, 2 out]
                        }
                        frame True {
                        }
                      }
                    }
                    frame #3 {
                      w308 = "\r"
                      # "Si un chip no està equalitzat,\nse li programa un PixelReg defecte"
                      # "default values for acquire"
                      # "PixelReg es crea segons I Leak"
                      n59 = local read "Layer ID list 2 (ordered)"() -> (w317:u32[])
                      n60 = local read "Layer ID list 1 (ordered)"() -> (w324:u32[])
                      n61 = for {
                        N: 100 -> [_]
                        tunnel: w326 -> [w370]
                        tunnel: [w367] -> w312 mode=concatenating
                        workers-P: _ -> [_]
                        w374 = u8 4  # bits 34, 35
                        # "100 x PixelReg"
                        n62 = Multiply(x=w370, y=w374) -> (x*y=w372:u8)
                        n63 = To Unsigned Long Integer(number=w372) -> (unsigned 32bit integer=w371:u32)
                        n64 = Add(x=u32 384, y=w371) -> (x+y=w368:u32)
                        n65 = Build Array(u32 671965161 ("Numeric"), w368) -> (w367:u32[])
                      }
                      n66 = call "Select PA gain.vi"() -> ("PA gain selected"=w306:u8)  [unwired: 5 in]
                      n67 = local read "Chip ID list 2"() -> (w316:u32[])
                      n68 = local read "Chip ID list 1"() -> (w323:u32[])
                      n69 = local read "All ID list 2"() -> (w318:u32[])
                      n70 = local read "All ID list 1"() -> (w325:u32[])
                      n71 = case shown="True" w319 {
                        tunnel: [w352 w366] -> w314
                        tunnel: w329 -> [_ w365]
                        tunnel: w328 -> [w352 w364]
                        tunnel: [w351 w361] -> w327
                        tunnel: w312 -> [_ w360]
                        tunnel: w311 -> [_ w359]
                        tunnel: w310 -> [_ w358]
                        tunnel: [_ w357] -> w309
                        tunnel: w325 -> [_ w354]
                        tunnel: w324 -> [_ w355]
                        tunnel: w323 -> [_ w356]
                        tunnel: w320 -> [w351 _]
                        tunnel: w306 -> [_ w353]
                        frame False {
                          # "Hardware 1 not enabled"
                        }
                        frame True {
                          # "Hardware 1 enabled"
                          n72 = call "PixelReg ProgramFromFile 2nPas.vi"("connection ID"=w365, "ACQ PxReg folder"=w358, "EQ folder path"=w359, "PixelReg (hex)"=w360, "All ID list"=w354, "Layer ID list"=w355, "Chip ID list"=w356, "error in (no error)"=w364, "PA gain"=w353) -> ("connection ID out"=w363:refnum<k5>, "done message"=w357:string, "All checks OK"=w361:bool, "error out (no error)"=w362:errorcluster)  [unwired: 2 in, 1 out]
                          n73 = call "CloseEthConnection.vi"("error in (no error)"=w362, "connection ID"=w363) -> ("error out"=w366:errorcluster)  [unwired: 9 in]
                        }
                      }
                      n74 = case shown="True" w320 {
                        tunnel: [w336 w350] -> w313
                        tunnel: w322 -> [_ w349]
                        tunnel: w321 -> [w336 w348]
                        tunnel: [w335 w345] -> w305
                        tunnel: w312 -> [_ w344]
                        tunnel: w311 -> [_ w343]
                        tunnel: w310 -> [_ w342]
                        tunnel: [_ w341] -> w303
                        tunnel: w318 -> [_ w338]
                        tunnel: w317 -> [_ w339]
                        tunnel: w316 -> [_ w340]
                        tunnel: w319 -> [w335 _]
                        tunnel: w306 -> [_ w337]
                        frame False {
                          # "Hardware 2 not enabled"
                        }
                        frame True {
                          # "Hardware 2 enabled"
                          n75 = call "PixelReg ProgramFromFile 2nPas.vi"("connection ID"=w349, "ACQ PxReg folder"=w342, "EQ folder path"=w343, "PixelReg (hex)"=w344, "All ID list"=w338, "Layer ID list"=w339, "Chip ID list"=w340, "error in (no error)"=w348, "PA gain"=w337) -> ("connection ID out"=w347:refnum<k5>, "done message"=w341:string, "All checks OK"=w345:bool, "error out (no error)"=w346:errorcluster)  [unwired: 2 in, 1 out]
                          n76 = call "CloseEthConnection.vi"("error in (no error)"=w346, "connection ID"=w347) -> ("error out"=w350:errorcluster)  [unwired: 9 in]
                        }
                      }
                      n77 = Merge Errors(w314, w313) -> (w315:errorcluster)
                      n78 = call <vilib>:"Simple Error Handler.vi"("error in (no error)"=w315) -> ()  [unwired: 4 in, 5 out]
                      n79 = Unbundle By Name(w315) -> ("status"=w330:bool)
                      n80 = Concatenate Strings "Concatenate Strings"(w304, w309, w308, w308, w307, w303) -> (w333:string)
                      n81 = Compound Arithmetic op=AND(invert w330, w327, w305) -> (w332:bool)
                      n82 = property on="Error tick" class="Bool (strict)"(reference=w331, "Value"=w330) -> ()  [unwired: 1 in, 2 out]
                      n83 = case shown="True" w332 {
                        tunnel: w333 -> [_ w376]
                        frame False {
                          # "error"
                        }
                        frame True {
                          # "OK x2"
                          n84 = call "MessageTimeOk.vi"("time (ms)"=5200, "missage"=w376) -> ()  [unwired: 4 in]
                        }
                      }
                    }
                  }
                }
              }
            }
            frame #1 {
              w379 = u32 0 ("Value")
              # "Mostra quina EQualització carrega"
              # "Llegeix HV final value from EQ loaded"
              # "Inicialitza variables 'actual time'"
              # "1) Inicialitzacions a la Adquisició. Ask for comments"
              n85 = flat-sequence {
                tunnel: w392 -> [w405]
                tunnel: [w404] -> w388
                tunnel: [w403] -> w386
                tunnel: w385 -> [w403]
                tunnel: [w409] -> w390
                tunnel: [w408] -> w389
                tunnel: w388 -> [w408]
                tunnel: w386 -> [w407]
                tunnel: [w412] -> w387
                tunnel: w390 -> [w412]
                tunnel: w389 -> [w411]
                frame #0 {
                  n86 = property on="Operation text" class="Str"(reference=w405, "Value"="Acquiring Pedestal...\nWrite comments for file.") -> (reference out=w404:refnum<vi>)  [unwired: 1 in, 1 out]
                }
                frame #1 {
                  # "ask for comments"
                  n87 = call "Acq_askComents.vi"("Folder path"=w407) -> ("Complete file path"=w409:path)  [unwired: 4 in]
                }
                frame #2 {
                  n88 = property on="Operation text" class="Str"(reference=w411, "Value"="Acquiring Pedestal...") -> ()  [unwired: 1 in, 2 out]
                }
              }
              n89 = property on="etapa2 Actual time" class="DigNum (strict)"(reference=w402, "Value"=w379) -> ()  [unwired: 1 in, 2 out]
              n90 = property on="etapa5 Actual time" class="DigNum (strict)"(reference=w400, "Value"=w379) -> ()  [unwired: 1 in, 2 out]
              n91 = property on="Events fets" class="DigNum (strict)"(reference=w380, "Value"=w379) -> ()  [unwired: 1 in, 2 out]
              n92 = property on="Events fets A" class="DigNum (strict)"(reference=w378, "Value"=w379) -> ()  [unwired: 1 in, 2 out]
              n93 = property on="Events fets B" class="DigNum (strict)"(reference=w377, "Value"=w379) -> ()  [unwired: 1 in, 2 out]
              n94 = property on="etapa3 Actual time" class="DigNum (strict)"(reference=w401, "Value"=w379) -> ()  [unwired: 1 in, 2 out]
              n95 = property on="HV parameters" class="Clust (strict)"(reference=w399) -> (reference out=w396:refnum<vi>, "Value"=w398:T5)  [unwired: 1 in, 1 out]
              n96 = property on="Stop ACQ button" class="Bool (strict)"(reference=w384, "Value"=FALSE, "DisabledEnum"=T4."Enabled" ("Disabled"), "Visible"=TRUE) -> ()  [unwired: 1 in, 2 out]
              n97 = in-place {
                in-place-border: w391 -> [w413]
                n98 = in-place-cluster #2(w398) -> ()  [unwired: 1 out]
                n99 = in-place-cluster #2("Final value"=w413) -> (w397:T5)
              }
              n100 = String To Path(string=w393) -> (path=w394:path)
              n101 = property class="Path"(reference="EQ folder path Refnum", "Value"=w394) -> ()  [unwired: 1 in, 2 out]
              n102 = property on="HV parameters" class="Clust (strict)"(reference=w396, "Value"=w397) -> ()  [unwired: 1 in, 2 out]
            }
            frame #2 {
              w415 = u32 0  # Comptador events per file
              w416 = u32 1  # first file sufix num.
              # "2) ADQUISICIÓ"
              n103 = while {
                tunnel: w440 -> [w470]
                tunnel: w439 -> [w469]
                tunnel: w438 -> [w468]
                tunnel: w437 -> [w467]
                tunnel: w436 -> [w466]
                tunnel: w435 -> [w465]
                tunnel: w434 -> [w464]
                tunnel: w433 -> [w463]
                tunnel: w432 -> [w462]
                tunnel: w431 -> [w461]
                tunnel: w430 -> [w460]
                tunnel: w429 -> [w459]
                tunnel: w428 -> [w458]
                tunnel: w420 -> [w457]
                tunnel: w427 -> [w456]
                tunnel: w426 -> [w455]
                tunnel: [w454] -> w425
                tunnel: w424 -> [w452]
                tunnel: w423 -> [w451]
                tunnel: w422 -> [w450]
                tunnel: w421 -> [w449]
                tunnel: w419 -> [w448]
                tunnel: w418 -> [w447]
                tunnel: w417 -> [w446]
                shift-right: [w443] -> _
                shift-left: w416 -> [w445]
                shift-right: [w442] -> _
                shift-left: w415 -> [w444]
                tunnel: w414 -> [w441]
                stop <- w453 stop-if-true
                n104 = stacked-sequence {
                  tunnel: w470 -> [_ _ w528 _ _ _ _]
                  tunnel: w469 -> [_ _ w530 _ _ _ _]
                  tunnel: w468 -> [w474 _ w529 _ _ _ _]
                  tunnel: w467 -> [_ _ _ w591 _ _ _]
                  tunnel: w466 -> [w473 _ _ w590 _ _ _]
                  tunnel: w465 -> [_ _ _ _ _ w812 _]
                  tunnel: w464 -> [_ _ _ _ _ w813 _]
                  tunnel: w463 -> [w472 _ _ _ _ w811 _]
                  tunnel: w462 -> [_ w486 _ _ w770 _ _]
                  tunnel: w461 -> [_ w479 _ _ w769 _ _]
                  tunnel: w460 -> [_ w482 _ w593 w768 _ _]
                  tunnel: w459 -> [_ w477 _ _ w767 _ _]
                  tunnel: w458 -> [_ w487 w527 w587 w762 w810 w861]
                  tunnel: w457 -> [_ w484 w526 _ w764 w809 _]
                  tunnel: w456 -> [_ _ _ w595 _ _ _]
                  tunnel: w455 -> [_ _ _ w594 _ _ _]
                  tunnel: [_ _ _ w592 _ _ _] -> w454
                  tunnel: [_ _ _ _ _ _ w860] -> w453
                  tunnel: w452 -> [_ _ _ w588 _ _ _]
                  tunnel: w451 -> [_ w476 w524 _ w763 w807 _]
                  tunnel: w450 -> [_ _ w522 _ _ w805 _]
                  tunnel: w449 -> [_ _ _ w586 w760 _ _]
                  tunnel: w448 -> [_ _ _ w585 _ _ _]
                  tunnel: w447 -> [_ _ _ w583 _ _ _]
                  tunnel: w446 -> [_ _ _ w584 _ _ _]
                  tunnel: w445 -> [_ _ _ w581 _ _ _]
                  tunnel: w444 -> [_ _ _ w580 _ _ _]
                  tunnel: [_ _ _ w578 _ _ _] -> w443
                  tunnel: [_ _ _ w579 _ _ _] -> w442
                  tunnel: w441 -> [_ _ _ w582 _ _ _]
                  frame #0 {
                    w471 = u8 0 ("ACQ-e2 barra")
                    # "Inicialitzacions a la iteració"
                    n105 = property on="etapa2 barra" class="Slide (strict)"(reference=w474, "Value"=w471) -> ()  [unwired: 1 in, 2 out]
                    n106 = property on="etapa3 barra" class="Slide (strict)"(reference=w473, "Value"=w471) -> ()  [unwired: 1 in, 2 out]
                    n107 = property on="etapa5 barra" class="Slide (strict)"(reference=w472, "Value"=w471) -> ()  [unwired: 1 in, 2 out]
                  }
                  frame #1 {
                    # "Etapa 1:  rampa pujada HV"
                    n108 = flat-sequence {
                      tunnel: w487 -> [w488]
                      tunnel: w486 -> [w493]
                      tunnel: [w496] -> w485
                      tunnel: w484 -> [w495]
                      tunnel: [w494] -> w483
                      tunnel: w482 -> [w494]
                      tunnel: [w493] -> w481
                      tunnel: [w492] -> w480
                      tunnel: w479 -> [w492]
                      tunnel: [w491] -> w478
                      tunnel: w477 -> [w491]
                      tunnel: w476 -> [w489]
                      tunnel: [w488] -> w475
                      frame #0 {
                        # "Desactiva busy per permetre\nmesura de temperatura\ndurant rampa HV i temps H"
                        n109 = property on="HV level" class="Slide (strict)"(reference=w493) -> ("Value"=w499:dbl)  [unwired: 1 in, 2 out]
                        n110 = property on="Stop ACQ" class="Bool (strict)"(reference=w488) -> ("Value"=w497:bool)  [unwired: 1 in, 2 out]
                        n111 = property on="busy = F" class="Bool (strict)"(reference=w489, "Value"=FALSE) -> ()  [unwired: 1 in, 2 out]
                        n112 = Not Equal To 0?(x=w499) -> (x != 0?=w498:bool)
                        n113 = Compound Arithmetic op=OR "OR"(w498, w497, invert w495) -> (w496:bool)
                      }
                    }
                    n114 = case shown="False" w485 {
                      tunnel: w480 -> [w507 _]
                      tunnel: w481 -> [w504 _]
                      tunnel: w483 -> [w503 _]
                      tunnel: w478 -> [w501 _]
                      tunnel: w475 -> [w500 _]
                      frame False {
                        n115 = flat-sequence {
                          tunnel: [w516] -> w510
                          tunnel: w507 -> [w521]
                          tunnel: [w519] -> w506
                          tunnel: [w518] -> w505
                          tunnel: w501 -> [w515]
                          frame #0 {
                            n116 = property on="HV parameters" class="Clust (strict)"(reference=w515) -> ("Value"=w516:T5)  [unwired: 1 in, 2 out]
                            n117 = property on="HV string" class="Str"(reference=w521, "Value"="HV ramping" ("HV String"), "Text.FontColor"=u32 15365376) -> (reference out=w519:refnum<vi>, error out=w518:errorcluster)  [unwired: 1 in]
                          }
                        }
                        n118 = call "HV_drive.vi"("Stop subVI Refnum"=w500, "HV level Refnum"=w504, "HV parameters"=w510) -> ("error out"=w509:errorcluster, "HV level (last value)"=w508:dbl)  [unwired: 1 in]
                        n119 = flat-sequence {
                          tunnel: w508 -> [_]
                          tunnel: w506 -> [w513]
                          tunnel: w505 -> [w512]
                          frame #0 {
                            n120 = property on="HV string" class="Str"(reference=w513, error in=w512, "Value"="HV presence!" ("HV String"), "Text.FontColor"=u32 16711680) -> ()  [unwired: 2 out]
                          }
                        }
                        n121 = Unbundle By Name(w509) -> ("status"=w502:bool)
                        n122 = call <vilib>:"Simple Error Handler.vi"("error in (no error)"=w509) -> ()  [unwired: 4 in, 5 out]
                        n123 = property on="Error tick" class="Bool (strict)"(reference=w503, "Value"=w502) -> ()  [unwired: 1 in, 2 out]
                      }
                      frame True {
                        # "executant aturada\no hi ha HV manual\no HV not enabled"
                      }
                    }
                  }
                  frame #2 {
                    # "Etapa 2:  temps inicial a HV_H"
                    n124 = flat-sequence {
                      tunnel: w530 -> [w537]
                      tunnel: w529 -> [w536]
                      tunnel: w528 -> [w535]
                      tunnel: w527 -> [w534]
                      tunnel: w526 -> [w533]
                      tunnel: [w532] -> w525
                      tunnel: w524 -> [w532]
                      tunnel: [w531] -> w523
                      tunnel: w522 -> [w531]
                      tunnel: w525 -> [w568]
                      tunnel: w523 -> [w567]
                      frame #0 {
                        n125 = case shown="True" w533 {
                          tunnel: w537 -> [_ w543]
                          tunnel: w536 -> [_ w541]
                          tunnel: w535 -> [_ w540]
                          tunnel: w534 -> [_ w539]
                          frame False {
                          }
                          frame True {
                            n126 = property on="etapa2 Actual time" class="DigNum (strict)"(reference=w543, "Value"=u32 0 ("ACQ-e2 Actual time")) -> (reference out=w542:refnum<vi>)  [unwired: 1 in, 1 out]
                            n127 = Tick Count (ms)() -> (millisecond timer value=w544:u32)
                            n128 = while {
                              tunnel: w544 -> [w563]
                              tunnel: w542 -> [w553]
                              tunnel: w540 -> [w552]
                              tunnel: w541 -> [w550]
                              tunnel: w539 -> [w546]
                              stop <- w548 stop-if-true
                              n129 = property on="etapa2 Waiting time" class="DigNum (strict)"(reference=w552) -> ("Value"=w551:u32)  [unwired: 1 in, 2 out]
                              n130 = Tick Count (ms)() -> (millisecond timer value=w564:u32)
                              n131 = property on="Stop ACQ" class="Bool (strict)"(reference=w546) -> ("Value"=w545:bool)  [unwired: 1 in, 2 out]
                              n132 = Subtract(x=w564, y=w563) -> (x-y=w562:u32)
                              n133 = Quotient & Remainder(x=w562, y=u32 1000) -> (floor(x/y)=w554:u32)  [unwired: 1 out]
                              n134 = Greater Or Equal?(x=w554, y=w551) -> (x >= y?=w547:bool)
                              n135 = To Double Precision Float(number=w554) -> (double precision float=w555:dbl)
                              n136 = To Double Precision Float(number=w551) -> (double precision float=w556:dbl)
                              n137 = property on="etapa2 Actual time" class="DigNum (strict)"(reference=w553, "Value"=w554) -> ()  [unwired: 1 in, 2 out]
                              n138 = Divide(x=w555, y=w556) -> (x/y=w559:dbl)
                              n139 = Or(x=w547, y=w545) -> (x .or. y?=w548:bool)
                              n140 = Multiply(x=w559, y=100.0) -> (x*y=w557:dbl)
                              n141 = To Unsigned Byte Integer(number=w557) -> (unsigned 8bit integer=w549:u8)
                              n142 = property on="etapa2 barra" class="Slide (strict)"(reference=w550, "Value"=w549) -> ()  [unwired: 1 in, 2 out]
                              n143 = Wait Until Next ms Multiple(millisecond multiple=u32 100) -> ()  [unwired: 1 out]
                            }
                          }
                        }
                      }
                      frame #1 {
                        # "Reactiva busy per procedir a l'adquisició"
                        n144 = flat-sequence {
                          tunnel: w568 -> [w573]
                          tunnel: w567 -> [w571]
                          tunnel: [w571] -> w569
                          tunnel: [w570] -> w565
                          tunnel: w569 -> [w575]
                          tunnel: [w574] -> w566
                          tunnel: w565 -> [w574]
                          tunnel: w566 -> [w576]
                          frame #0 {
                            n145 = property on="busy = T" class="Bool (strict)"(reference=w573, "Value"=TRUE) -> (reference out=w570:refnum<vi>)  [unwired: 1 in, 1 out]
                          }
                          frame #1 {
                            n146 = Wait (ms)(milliseconds to wait=w575) -> ()  [unwired: 1 out]
                          }
                          frame #2 {
                            n147 = property on="busy = T" class="Bool (strict)"(reference=w576, "Value"=TRUE) -> ()  [unwired: 1 in, 2 out]
                          }
                        }
                      }
                    }
                  }
                  frame #3 {
                    # "Etapa 3:  adquisició Pedestal"
                    n148 = property on="Stop ACQ button" class="Bool (strict)"(reference=w587) -> ("Value"=w589:bool)  [unwired: 1 in, 2 out]
                    n149 = case shown="False" w589 {
                      tunnel: w595 -> [w606 _]
                      tunnel: w594 -> [w613 _]
                      tunnel: w593 -> [w616 _]
                      tunnel: w587 -> [w615 _]
                      tunnel: [w607 _] -> w592
                      tunnel: w591 -> [w609 _]
                      tunnel: w590 -> [w610 _]
                      tunnel: w588 -> [w608 _]
                      tunnel: w586 -> [w605 _]
                      tunnel: w585 -> [w603 _]
                      tunnel: w584 -> [w602 _]
                      tunnel: w583 -> [w601 _]
                      tunnel: w582 -> [w600 _]
                      tunnel: w581 -> [w598 w759]
                      tunnel: w580 -> [w599 w758]
                      tunnel: [w597 w758] -> w579
                      tunnel: [w596 w759] -> w578
                      frame False {
                        # "si no hi ha Stop ordenat, adquireix"
                        n150 = local read "Addresses Cluster"() -> (w614:T1)
                        n151 = Array Size(array=w603) -> (size(s)=w604:i32)
                        n152 = in-place "Conversion of DTP: ms to comptes" {
                          n153 = in-place-cluster #3("ACQ Parameters (cluster)") -> ("DTP period"=w752:u32)
                          n154 = To Double Precision Float(number=w752) -> (double precision float=w753:dbl)
                          n155 = Divide(x=w753, y=2.5e-05) -> (x/y=w756:dbl)
                          n156 = Decrement(x=w756) -> (x-1=w755:dbl)
                          n157 = To Unsigned Long Integer(number=w755) -> (unsigned 32bit integer=w754:u32)
                          n158 = in-place-cluster #3("DTP period"=w754) -> (w621:T2)
                        }
                        n159 = property class="DigNum (strict)"(reference="Events to acquire Refnum") -> ("Value"=w617:u32)  [unwired: 1 in, 2 out]
                        n160 = Cluster To Array(cluster=w621) -> (array=w611:u32[])
                        n161 = Bundle(TRUE, "Value"=w617) -> (w612:cluster{bool, "Value":u32})  [unwired: 1 in]
                        n162 = for {
                          tunnel: w616 -> [w645]
                          tunnel: w615 -> [w634]
                          tunnel: w614 -> [w644]
                          tunnel: w613 -> [w643]
                          tunnel: w612 -> [w642]
                          tunnel: w611 -> [w641]
                          tunnel: w610 -> [w640]
                          tunnel: w609 -> [w639]
                          tunnel: w608 -> [w638]
                          tunnel: [w637] -> w607
                          tunnel: w606 -> [w636]
                          tunnel: w605 -> [w635]
                          tunnel: w603 -> [w631] mode=indexing
                          tunnel: w604 -> [w629]
                          tunnel: w602 -> [w628]
                          tunnel: w601 -> [w627]
                          tunnel: w600 -> [w626]
                          shift-right: [w622] -> w597
                          shift-left: w599 -> [w624]
                          shift-right: [w623] -> w596
                          shift-left: w598 -> [w625]
                          i -> [w630]
                          stop <- w633 stop-if-true
                          n163 = property on="Stop ACQ button" class="Bool (strict)"(reference=w634) -> ("Value"=w633:bool)  [unwired: 1 in, 2 out]
                          n164 = call "GlobalRegEd px_triggerEN.vi"("Pixel number"=w631, "Global Reg (default)"=w626) -> ("Global Regster (U32)"=w632:u32[])  [unwired: 3 in]
                          n165 = stacked-sequence {
                            tunnel: w645 -> [_ w662 w716 _]
                            tunnel: w634 -> [_ _ w715 _]
                            tunnel: w644 -> [_ w672 w714 _]
                            tunnel: w643 -> [_ _ w711 w747]
                            tunnel: w642 -> [_ _ w726 _]
                            tunnel: w641 -> [_ _ w725 _]
                            tunnel: w640 -> [_ _ w724 _]
                            tunnel: w639 -> [_ _ w723 _]
                            tunnel: w636 -> [_ _ w722 _]
                            tunnel: w638 -> [w649 _ w721 _]
                            tunnel: [_ _ w717 _] -> w637
                            tunnel: w632 -> [_ w666 _ _]
                            tunnel: w635 -> [w656 _ _ _]
                            tunnel: w631 -> [w651 _ _ _]
                            tunnel: w630 -> [w654 _ _ _]
                            tunnel: w629 -> [w652 _ _ _]
                            tunnel: w628 -> [w646 _ w712 _]
                            tunnel: w627 -> [w647 _ w713 _]
                            tunnel: w625 -> [_ _ _ w751]
                            tunnel: w624 -> [_ _ _ w750]
                            tunnel: [_ _ _ w749] -> w623
                            tunnel: [_ _ _ w748] -> w622
                            frame #0 {
                              w648 = u32 0 ("Value")
                              # "operation text: <px>"
                              n166 = Increment(x=w654) -> (x+1=w653:i32)
                              n167 = property on="Events fets (per pixel)" class="DigNum (strict)"(reference=w649, "Value"=w648) -> ()  [unwired: 1 in, 2 out]
                              n168 = property on="Events fets A" class="DigNum (strict)"(reference=w647, "Value"=w648) -> ()  [unwired: 1 in, 2 out]
                              n169 = property on="Events fets B" class="DigNum (strict)"(reference=w646, "Value"=w648) -> ()  [unwired: 1 in, 2 out]
                              n170 = Format Into String "Format Into String"(format string="Acquisition Pedestal...\n(%d/%d) Central px: %d", w653, w652, w651) -> (resulting string=w650:string)  [unwired: 2 in, 1 out]
                              n171 = property on="operation text" class="Str"(reference=w656, "Value"=w650) -> ()  [unwired: 1 in, 2 out]
                            }
                            frame #1 {
                              w667 = u32 65535  # LayerID & ChipID
                              # "0) Program Glogal Reg <px>"
                              n172 = Unbundle By Name(w672) -> ("ENA1"=w668:bool, "IP address 1"=w669:string, "ENA2"=w670:bool, "IP address 2"=w671:string)
                              n173 = case shown="True" w668 {
                                tunnel: w667 -> [_ w702]
                                tunnel: [_ w705] -> w658
                                tunnel: [w697 w704] -> w660
                                tunnel: w666 -> [_ w703]
                                tunnel: w669 -> [_ w701]
                                tunnel: w670 -> [w697 _]
                                tunnel: [_ w698] -> w664
                                frame False {
                                # "Hardware 1 not enabled"
                                }
                                frame True {
                                # "Hardware 1 enabled"
                                n174 = call "OpenEthConnection.vi"("Port"=u16 80, "IP address"=w701) -> ("error out"=w709:errorcluster, "connection ID out"=w710:refnum<k5>)  [unwired: 7 in, 1 out]
                                n175 = call "ProgramGlobalReg.vi"("Global Reg"=w703, "error in (no error)"=w709, "ChipID"=w702, "LayerID"=w702, "connection ID"=w710) -> ("error out"=w699:errorcluster, "OK?"=w704:bool, "connection ID out"=w700:refnum<k5>, "Program done"=w707:string[])  [unwired: 2 in, 1 out]
                                n176 = Index Array "Index Array"(array=w707, index=1) -> (element=w705:string)
                                n177 = call "CloseEthConnection.vi"("error in (no error)"=w699, "connection ID"=w700) -> ("error out"=w698:errorcluster)  [unwired: 9 in]
                                }
                              }
                              n178 = case shown="True" w670 {
                                tunnel: w667 -> [_ w688]
                                tunnel: [_ w691] -> w657
                                tunnel: [w683 w690] -> w659
                                tunnel: w666 -> [_ w689]
                                tunnel: w671 -> [_ w687]
                                tunnel: w668 -> [w683 _]
                                tunnel: [_ w684] -> w663
                                frame False {
                                # "Hardware 2 not enabled"
                                }
                                frame True {
                                # "Hardware 2 enabled"
                                n179 = call "OpenEthConnection.vi"("Port"=u16 80, "IP address"=w687) -> ("error out"=w695:errorcluster, "connection ID out"=w696:refnum<k5>)  [unwired: 7 in, 1 out]
                                n180 = call "ProgramGlobalReg.vi"("Global Reg"=w689, "error in (no error)"=w695, "ChipID"=w688, "LayerID"=w688, "connection ID"=w696) -> ("error out"=w685:errorcluster, "OK?"=w690:bool, "connection ID out"=w686:refnum<k5>, "Program done"=w693:string[])  [unwired: 2 in, 1 out]
                                n181 = Index Array "Index Array"(array=w693, index=1) -> (element=w691:string)
                                n182 = call "CloseEthConnection.vi"("error in (no error)"=w685, "connection ID"=w686) -> ("error out"=w684:errorcluster)  [unwired: 9 in]
                                }
                              }
                              n183 = Merge Errors(w664, w663) -> (w665:errorcluster)
                              n184 = call <vilib>:"Simple Error Handler.vi"("error in (no error)"=w665) -> ()  [unwired: 4 in, 5 out]
                              n185 = Unbundle By Name(w665) -> ("status"=w661:bool)
                              n186 = disable-structure shown="Disabled" {
                                disable-tunnel: w661 -> [w680 _]
                                disable-tunnel: w660 -> [w679 _]
                                disable-tunnel: w659 -> [w678 _]
                                disable-tunnel: w658 -> [w677 _]
                                disable-tunnel: w657 -> [w675 _]
                                frame Disabled {
                                w676 = "\r"
                                n187 = Concatenate Strings "Concatenate Strings"(w677, w676, w676, w675) -> (w673:string)
                                n188 = Compound Arithmetic op=AND "AND"(invert w680, w679, w678) -> (w674:bool)
                                n189 = case shown="True" w674 {
                                tunnel: w673 -> [_ w682]
                                frame False {
                                # "error"
                                }
                                frame True {
                                # "OK x1"
                                n190 = call "MessageTimeOk.vi"("time (ms)"=1000, "missage"=w682) -> ()  [unwired: 4 in]
                                }
                                }
                                }
                                frame Enabled {
                                }
                              }
                              n191 = property on="Error tick" class="Bool (strict)"(reference=w662, "Value"=w661) -> ()  [unwired: 1 in, 2 out]
                            }
                            frame #2 {
                              # "1) Acquire Pedestal <px>"
                              n192 = call "subop_x2_Acquisition.vi"("ACQ stop by events"=w726, "ACQ parameters"=w725, "events fets A Refnum"=w713, "events fets B Refnum"=w712, "Base file path"=w711, "Addresses Cluster"=w714, "Stop ACQ button Refnum"=w715, "ACQ barra Refnum"=w724, "Actual time Refnum"=w723, "Acquisition time Refnum"=w722, "Total events Refnum"=w721) -> ("ACQ WatchDog timeout"=w717:bool, "ACQ Answer 1i2"=w718:string, "error out comm"=w720:errorcluster, "error out file"=w719:errorcluster)  [unwired: 12 in, 1 out]
                              n193 = flat-sequence {
                                tunnel: w717 -> [w731]
                                tunnel: w715 -> [w730]
                                tunnel: w717 -> [w735]
                                frame #0 {
                                n194 = case shown="True" w731 {
                                tunnel: w730 -> [_ w734]
                                frame False {
                                }
                                frame True {
                                # "Watchdog: stop execution"
                                n195 = property on="Stop ACQ button" class="Bool (strict)"(reference=w734, "Value"=TRUE, "DisabledEnum"=T4."Disabled" ("Disabled")) -> ()  [unwired: 1 in, 2 out]
                                }
                                }
                                }
                                frame #1 {
                                n196 = case shown="True" w735 {
                                frame False {
                                }
                                frame True {
                                n197 = One Button Dialog(message="Acquisition WatchDog timeout.") -> ()  [unwired: 1 in, 1 out]
                                }
                                }
                                }
                              }
                              n198 = Merge Errors(w720, w719) -> (w729:errorcluster)
                              n199 = call <vilib>:"Simple Error Handler.vi"("error in (no error)"=w729) -> ()  [unwired: 4 in, 5 out]
                              n200 = Unbundle By Name(w729) -> ("status"=w728:bool)
                              n201 = property on="Error tick" class="Bool (strict)"(reference=w716, "Value"=w728) -> ()  [unwired: 1 in, 2 out]
                              n202 = Or(x=w719, y=w717) -> (x .or. y?=w727:bool)
                              n203 = case shown="False" w727 {
                                tunnel: w718 -> [w737 _]
                                frame False {
                                # "No hi ha errors file"
                                n204 = Concatenate Strings(w737, "\r", "The file have been saved.") -> (w740:string)
                                n205 = call "MessageTimeOk.vi"("time (ms)"=800, "missage"=w740) -> ()  [unwired: 4 in]
                                }
                                frame True {
                                # "Algun error"
                                }
                              }
                            }
                            frame #3 {
                              # "2) Merge temp files"
                              n206 = local read "Chip ID list 1"() -> (w745:u32[])
                              n207 = local read "Chip ID list 2"() -> (w744:u32[])
                              n208 = local read "Addresses Cluster"() -> (w746:T1)
                              n209 = To Unsigned Word Integer(number=w745) -> (unsigned 16bit integer=w743:u16[])
                              n210 = To Unsigned Word Integer(number=w744) -> (unsigned 16bit integer=w742:u16[])
                              n211 = call "ACQ PostProces1.vi"("ACQ full DATA file path"=w747, "Addresses Cluster"=w746, "Chip ID list 2"=w742, "Chip ID list 1"=w743, "events per file in"=w750, "file sufix num. in"=w751) -> ("events per file out"=w748:u32, "file sufix num. out"=w749:u32)  [unwired: 2 in, 2 out]
                            }
                          }
                        }
                      }
                      frame True {
                        # "Stop ordenat"
                      }
                    }
                  }
                  frame #4 {
                    # "Tant si hi ha Stop adquisició ordenat com si no, executa rampa baixada HV"
                    # "Etapa 4:  rampa bajada HV"
                    n212 = flat-sequence {
                      tunnel: w764 -> [w774]
                      tunnel: w763 -> [w775]
                      tunnel: [w774] -> w761
                      tunnel: w760 -> [w773]
                      frame #0 {
                        # "Desactiva busy per permetre\nmesura de temperatura\ndurant rampa HV i temps L"
                        n213 = property on="busy = F" class="Bool (strict)"(reference=w775, "Value"=FALSE) -> ()  [unwired: 1 in, 2 out]
                        n214 = property class="Str"(reference=w773, "Value"="Acquiring Pedestal...") -> ()  [unwired: 1 in, 2 out]
                      }
                    }
                    n215 = property on="HV level" class="Slide (strict)"(reference=w770) -> ("Value"=w771:dbl)  [unwired: 1 in, 2 out]
                    n216 = Not Equal To 0?(x=w771) -> (x != 0?=w766:bool)
                    n217 = And(x=w766, y=w761) -> (x .and. y?=w765:bool)
                    n218 = case shown="True" w765 {
                      tunnel: w770 -> [_ w781]
                      tunnel: w769 -> [_ w780]
                      tunnel: w768 -> [_ w779]
                      tunnel: w767 -> [_ w778]
                      tunnel: w762 -> [_ w777]
                      frame False {
                        # "HV = 0,   no cal baixada"
                      }
                      frame True {
                        n219 = flat-sequence {
                          tunnel: [w798] -> w782
                          tunnel: w780 -> [w804]
                          tunnel: [w802] -> w785
                          tunnel: [w801] -> w786
                          tunnel: w778 -> [w799]
                          frame #0 {
                            n220 = property on="HV parameters" class="Clust (strict)"(reference=w799) -> ("Value"=w798:T5)  [unwired: 1 in, 2 out]
                            n221 = property on="HV string" class="Str"(reference=w804, "Value"="HV ramping" ("HV String"), "Text.FontColor"=u32 15365376) -> (reference out=w802:refnum<vi>, error out=w801:errorcluster)  [unwired: 1 in]
                          }
                        }
                        n222 = call "HV_drive.vi"("Stop subVI Refnum"=w777, "HV level Refnum"=w781, "HV parameters"=w782) -> ("error out"=w783:errorcluster, "HV level (last value)"=w784:dbl)  [unwired: 1 in]
                        n223 = flat-sequence {
                          tunnel: w784 -> [w790]
                          tunnel: w785 -> [w797]
                          tunnel: w786 -> [w796]
                          frame #0 {
                            n224 = Equal To 0?(x=w790) -> (x = 0?=w795:bool)
                            n225 = Select(t="HV off", s=w795, f="HV presence!") -> (s? t:f=w789:string)
                            n226 = Select(t=u32 42533, s=w795, f=u32 16711680) -> (s? t:f=w788:u32)
                            n227 = property on="HV string" class="Str"(reference=w797, error in=w796, "Value"=w789, "Text.FontColor"=w788) -> ()  [unwired: 2 out]
                          }
                        }
                        n228 = Unbundle By Name(w783) -> ("status"=w787:bool)
                        n229 = call <vilib>:"Simple Error Handler.vi"("error in (no error)"=w783) -> ()  [unwired: 4 in, 5 out]
                        n230 = property on="Error tick" class="Bool (strict)"(reference=w779, "Value"=w787) -> ()  [unwired: 1 in, 2 out]
                      }
                    }
                  }
                  frame #5 {
                    # "Etapa 5:  temps final a HV_L"
                    n231 = flat-sequence {
                      tunnel: w813 -> [w820]
                      tunnel: w812 -> [w819]
                      tunnel: w811 -> [w818]
                      tunnel: w810 -> [w817]
                      tunnel: w809 -> [w816]
                      tunnel: [w815] -> w808
                      tunnel: w807 -> [w815]
                      tunnel: [w814] -> w806
                      tunnel: w805 -> [w814]
                      tunnel: w808 -> [w854]
                      tunnel: w806 -> [w853]
                      frame #0 {
                        n232 = disable-structure shown="Disabled" {
                          disable-tunnel: w820 -> [w825 _]
                          disable-tunnel: w819 -> [w824 _]
                          disable-tunnel: w818 -> [w823 _]
                          disable-tunnel: w817 -> [w822 _]
                          disable-tunnel: w816 -> [w821 _]
                          frame Disabled {
                            n233 = case shown="True" w821 {
                              tunnel: w825 -> [_ w832]
                              tunnel: w824 -> [_ w829]
                              tunnel: w823 -> [_ w828]
                              tunnel: w822 -> [_ w827]
                              frame False {
                              }
                              frame True {
                                n234 = property on="etapa5 Actual time" class="DigNum (strict)"(reference=w832, "Value"=u32 0 ("ACQ-e2 Actual time")) -> (reference out=w830:refnum<vi>)  [unwired: 1 in, 1 out]
                                n235 = Tick Count (ms)() -> (millisecond timer value=w831:u32)
                                n236 = while {
                                tunnel: w831 -> [w851]
                                tunnel: w830 -> [w841]
                                tunnel: w829 -> [w840]
                                tunnel: w828 -> [w838]
                                tunnel: w827 -> [w834]
                                stop <- w836 stop-if-true
                                # "et5: temps final a HV_L"
                                n237 = property on="etapa5 Waiting time" class="DigNum (strict)"(reference=w840) -> ("Value"=w839:u32)  [unwired: 1 in, 2 out]
                                n238 = Tick Count (ms)() -> (millisecond timer value=w852:u32)
                                n239 = property on="Stop ACQ" class="Bool (strict)"(reference=w834) -> ("Value"=w833:bool)  [unwired: 1 in, 2 out]
                                n240 = Subtract(x=w852, y=w851) -> (x-y=w850:u32)
                                n241 = Quotient & Remainder(x=w850, y=u32 1000) -> (floor(x/y)=w842:u32)  [unwired: 1 out]
                                n242 = Greater Or Equal?(x=w842, y=w839) -> (x >= y?=w835:bool)
                                n243 = To Double Precision Float(number=w842) -> (double precision float=w843:dbl)
                                n244 = To Double Precision Float(number=w839) -> (double precision float=w844:dbl)
                                n245 = property on="etapa5 Actual time" class="DigNum (strict)"(reference=w841, "Value"=w842) -> ()  [unwired: 1 in, 2 out]
                                n246 = Or(x=w835, y=w833) -> (x .or. y?=w836:bool)
                                n247 = Divide(x=w843, y=w844) -> (x/y=w847:dbl)
                                n248 = Multiply(x=w847, y=100.0) -> (x*y=w845:dbl)
                                n249 = To Unsigned Byte Integer(number=w845) -> (unsigned 8bit integer=w837:u8)
                                n250 = property on="etapa5 barra" class="Slide (strict)"(reference=w838, "Value"=w837) -> ()  [unwired: 1 in, 2 out]
                                n251 = Wait Until Next ms Multiple(millisecond multiple=u32 100) -> ()  [unwired: 1 out]
                                }
                              }
                            }
                          }
                          frame Enabled {
                          }
                        }
                      }
                      frame #1 {
                        # "Reactiva busy per seguir amb la seqüència"
                        n252 = flat-sequence {
                          tunnel: w854 -> [w858]
                          tunnel: w853 -> [w856]
                          tunnel: [w856] -> w855
                          tunnel: w855 -> [w859]
                          frame #0 {
                            n253 = property on="busy = T" class="Bool (strict)"(reference=w858, "Value"=TRUE) -> ()  [unwired: 1 in, 2 out]
                          }
                          frame #1 {
                            n254 = Wait (ms)(milliseconds to wait=w859) -> ()  [unwired: 1 out]
                          }
                        }
                      }
                    }
                  }
                  frame #6 {
                    # "aturar adquisició?"
                    n255 = disable-structure shown="Enabled" {
                      disable-tunnel: w861 -> [w863 _]
                      disable-tunnel: [w862 w864] -> w860
                      frame Disabled {
                        n256 = property on="Stop ACQ" class="Bool (strict)"(reference=w863) -> ("Value"=w862:bool)  [unwired: 1 in, 2 out]
                      }
                      frame Enabled {
                        w864 = TRUE  # only one HV run
                      }
                    }
                  }
                }
              }
            }
            frame #3 {
              # "3) Finalització a l'adquisició. Restaura Global Registers."
              n257 = flat-sequence {
                tunnel: w870 -> [w873]
                tunnel: [w873] -> w869
                tunnel: w868 -> [w872]
                tunnel: w869 -> [w875]
                tunnel: w865 -> [w874]
                tunnel: w867 -> [w924]
                tunnel: w866 -> [w923]
                frame #0 {
                  n258 = property class="Str"(reference=w872, "Value"="Acquiring Pedestal...\nRestoring Global Regs.") -> ()  [unwired: 1 in, 2 out]
                }
                frame #1 {
                  w880 = "\r"
                  w888 = u32 65535  # LayerID & ChipID
                  # "Restaura Global Registers."
                  n259 = local read "Addresses Cluster"() -> (w876:T1)
                  n260 = Unbundle By Name(w876) -> ("ENA1"=w889:bool, "IP address 1"=w890:string, "ENA2"=w891:bool, "IP address 2"=w892:string)
                  n261 = case shown="True" w889 {
                    tunnel: w888 -> [_ w914]
                    tunnel: [_ w917] -> w881
                    tunnel: [w909 w916] -> w883
                    tunnel: w874 -> [_ w915]
                    tunnel: w890 -> [_ w913]
                    tunnel: w891 -> [w909 _]
                    tunnel: [_ w910] -> w886
                    frame False {
                      # "Hardware 1 not enabled"
                    }
                    frame True {
                      # "Hardware 1 enabled"
                      n262 = call "OpenEthConnection.vi"("Port"=u16 80, "IP address"=w913) -> ("error out"=w921:errorcluster, "connection ID out"=w922:refnum<k5>)  [unwired: 7 in, 1 out]
                      n263 = call "ProgramGlobalReg.vi"("Global Reg"=w915, "error in (no error)"=w921, "ChipID"=w914, "LayerID"=w914, "connection ID"=w922) -> ("error out"=w911:errorcluster, "OK?"=w916:bool, "connection ID out"=w912:refnum<k5>, "Program done"=w919:string[])  [unwired: 2 in, 1 out]
                      n264 = Index Array "Index Array"(array=w919, index=1) -> (element=w917:string)
                      n265 = call "CloseEthConnection.vi"("error in (no error)"=w911, "connection ID"=w912) -> ("error out"=w910:errorcluster)  [unwired: 9 in]
                    }
                  }
                  n266 = case shown="True" w891 {
                    tunnel: w888 -> [_ w900]
                    tunnel: [_ w903] -> w879
                    tunnel: [w895 w902] -> w882
                    tunnel: w874 -> [_ w901]
                    tunnel: w892 -> [_ w899]
                    tunnel: w889 -> [w895 _]
                    tunnel: [_ w896] -> w885
                    frame False {
                      # "Hardware 2 not enabled"
                    }
                    frame True {
                      # "Hardware 2 enabled"
                      n267 = call "OpenEthConnection.vi"("Port"=u16 80, "IP address"=w899) -> ("error out"=w907:errorcluster, "connection ID out"=w908:refnum<k5>)  [unwired: 7 in, 1 out]
                      n268 = call "ProgramGlobalReg.vi"("Global Reg"=w901, "error in (no error)"=w907, "ChipID"=w900, "LayerID"=w900, "connection ID"=w908) -> ("error out"=w897:errorcluster, "OK?"=w902:bool, "connection ID out"=w898:refnum<k5>, "Program done"=w905:string[])  [unwired: 2 in, 1 out]
                      n269 = Index Array "Index Array"(array=w905, index=1) -> (element=w903:string)
                      n270 = call "CloseEthConnection.vi"("error in (no error)"=w897, "connection ID"=w898) -> ("error out"=w896:errorcluster)  [unwired: 9 in]
                    }
                  }
                  n271 = Merge Errors(w886, w885) -> (w887:errorcluster)
                  n272 = call <vilib>:"Simple Error Handler.vi"("error in (no error)"=w887) -> ()  [unwired: 4 in, 5 out]
                  n273 = Unbundle By Name(w887) -> ("status"=w884:bool)
                  n274 = Concatenate Strings "Concatenate Strings"(w881, w880, w880, w879) -> (w877:string)
                  n275 = Compound Arithmetic op=AND "AND"(invert w884, w883, w882) -> (w878:bool)
                  n276 = property on="Error tick" class="Bool (strict)"(reference=w875, "Value"=w884) -> ()  [unwired: 1 in, 2 out]
                  n277 = case shown="True" w878 {
                    tunnel: w877 -> [_ w894]
                    frame False {
                      # "error"
                    }
                    frame True {
                      # "OK x1"
                      n278 = call "MessageTimeOk.vi"("time (ms)"=1000, "missage"=w894) -> ()  [unwired: 4 in]
                    }
                  }
                }
                frame #2 {
                  w925 = FALSE ("Value")
                  # "Desactiva busy per permetre\nmesura de temperatura\ndurant ACQ data viewer."
                  n279 = property on="Stop ACQ button" class="Bool (strict)"(reference=w924, "Visible"=w925, "Value"=w925, "DisabledEnum"=T4."Enabled" ("Disabled")) -> ()  [unwired: 1 in, 2 out]
                  n280 = property on="busy = F" class="Bool (strict)"(reference=w923, "Value"=FALSE) -> ()  [unwired: 1 in, 2 out]
                }
              }
            }
            frame #4 {
              # "4) Open DATA viewer"
              n281 = local read "ACQ Parameters (cluster)"() -> (w941:T2)
              n282 = property on="ACQ events fets" class="DigNum (strict)"(reference=w932) -> ("Value"=w943:u32)  [unwired: 1 in, 2 out]
              n283 = property on="etapa2 Waiting time (s)" class="DigNum (strict)"(reference=w928) -> ("Value"=w940:u32)  [unwired: 1 in, 2 out]
              n284 = property on="etapa5 Waiting time (s)" class="DigNum (strict)"(reference=w929) -> ("Value"=w939:u32)  [unwired: 1 in, 2 out]
              n285 = property on="Acquisition time (s)" class="DigNum (strict)"(reference=w930) -> ("Value"=w938:u32)  [unwired: 1 in, 2 out]
              n286 = local read "GbReg params"() -> (w944:u8[])
              n287 = property on="HV parameters" class="Clust (strict)"(reference=w931) -> ("Value"=w942:T5)  [unwired: 1 in, 2 out]
              n288 = Index Array "Index Array"(array=w944) -> (element #1=w937:u8, element #2=w936:u8)  [unwired: 2 in]
              n289 = call "Grava_conditionsACQ.vi"("ACQ Parameters (cluster)"=w941, "HV parameters"=w942, "ACQ events fets"=w943, "EQ folder path"=w933, "ACQ folder path"=w934, "EQ loaded?"=w935, "etapa2 Waiting time (s)"=w940, "ACQ anVref low"=w937, "Acquisition time (s)"=w938, "ACQ GbTHLD"=w936, "etapa5 Waiting time (s)"=w939) -> ()  [unwired: 9 in]
              n290 = disable-structure shown="Disabled" {
                disable-tunnel: w948 -> [w953 _]
                disable-tunnel: w947 -> [w952 _]
                disable-tunnel: w946 -> [w951 _]
                disable-tunnel: w932 -> [w950 _]
                disable-tunnel: w945 -> [w949 _]
                frame Disabled {
                  n291 = case shown="False" w953 {
                    tunnel: w952 -> [w961 _]
                    tunnel: w951 -> [w960 _]
                    tunnel: w950 -> [w959 _]
                    tunnel: w949 -> [w955 _]
                    frame False {
                      # "No hi ha timeout: obre DATA viewer"
                      n292 = flat-sequence {
                        tunnel: w959 -> [w967]
                        tunnel: w960 -> [w968]
                        tunnel: w961 -> [w969]
                        tunnel: [w969] -> w958
                        tunnel: [w968] -> w957
                        tunnel: [w967] -> w956
                        tunnel: w955 -> [w966]
                        tunnel: [w962] -> w954
                        tunnel: w958 -> [w977]
                        tunnel: w957 -> [w981]
                        tunnel: w956 -> [w980]
                        tunnel: w954 -> [w978]
                        frame #0 {
                          n293 = local read "Chip ID list 1"() -> (w964:u32[])
                          n294 = local read "Chip ID list 2"() -> (w963:u32[])
                          n295 = property on="Operation text" class="Str"(reference=w966, "Value"="Acquiring...\nData viewer open") -> ()  [unwired: 1 in, 2 out]
                          n296 = Build Array (concatenate) "Concatenate"(w964, w963) -> (w962:u32[])
                        }
                        frame #1 {
                          n297 = Strip Path(path=w977) -> (stripped path=w976:path)  [unwired: 1 out]
                          n298 = List Folder(path=w976, pattern="*.dat") -> (filenames=w974:string[])  [unwired: 2 in, 3 out]
                          n299 = Array Size(array=w974) -> (size(s)=w973:i32)
                          n300 = for {
                            N: w973 -> [_]
                            tunnel: w978 -> [w995]
                            tunnel: w977 -> [w997]
                            shift-right: [w999] -> _
                            shift-left: w973 -> [w1000]
                            tunnel: [w998] -> w971
                            tunnel: [w996] -> w972
                            tunnel: [w995] -> w970
                            n301 = To Unsigned Long Integer(number=w1000) -> (unsigned 32bit integer=w1001:u32)
                            n302 = Decrement(x=w1000) -> (x-1=w999:i32)
                            n303 = call "Grava_summaryACQ.vi"("sufix number"=w1001, "ChipID list"=w995, "ACQ full DATA file path"=w997) -> ("quants events per chip"=w998:u32[], "suffixed file path"=w996:path)  [unwired: 1 in]
                          }
                          n304 = property class="DigNum (strict)"(reference=w980) -> ("Value"=w979:u32)  [unwired: 1 in, 2 out]
                          n305 = disable-structure shown="Disabled" {
                            disable-tunnel: w981 -> [w987 _]
                            disable-tunnel: w979 -> [w986 _]
                            disable-tunnel: w973 -> [w985 _]
                            disable-tunnel: w972 -> [w984 _]
                            disable-tunnel: w971 -> [w983 _]
                            disable-tunnel: w970 -> [w982 _]
                            frame Disabled {
                              # "No obrir per falta de memòria en WinXP"
                              n306 = case shown="1" w985 {
                                tunnel: w987 -> [_ w994]
                                tunnel: w986 -> [_ w993]
                                tunnel: w984 -> [_ w992]
                                tunnel: w983 -> [_ w990]
                                tunnel: w982 -> [_ w991]
                                frame Default {
                                # "Empty file path\nEmpty ChipID list"
                                # "to choose ACQ file"
                                n307 = call "ACQ_Data_viewer (Module).vi"("ACQ full DATA file path"=path "", "ChipID list"=u32[] []) -> ()  [unwired: 14 in]
                                }
                                frame 1 {
                                # "only one ACQ file"
                                n308 = call "ACQ_Data_viewer (Module).vi"("ACQ full DATA file path"=w992, "ChipID list"=w991, "quants events per chip"=w990, "ID summary"=w994, "ACQ events fets"=w993) -> ()  [unwired: 11 in]
                                }
                              }
                            }
                            frame Enabled {
                            }
                          }
                        }
                      }
                    }
                    frame True {
                    }
                  }
                }
                frame Enabled {
                }
              }
            }
          }
        }
      }
    }
    frame True {
      # "connection not working"
      n309 = property on="Error tick" class="Bool (strict)"(reference=w1002, "Value"=w1003) -> ()  [unwired: 1 in, 2 out]
      n310 = One Button Dialog(message="The connection is NOT WORKING.\n\nCheck the wiring connection and the IP address.") -> ()  [unwired: 1 in, 1 out]
    }
  }
  "Folder path: acquisition reports" <- w1
